vi "Gymkhana.vi"() -> ()   [LabVIEW 2020]
uses:
  Control/GymkhanaBestRecordIndicator.ctl
  Control/GymkhanaCurrentRecordIndicator.ctl
  Control/GymkhanaSubLoopState.ctl
  Control/GymkhanaFlag.ctl
  CommonControl/Flag.ctl
  Control/GymkhanaMainLoopState.ctl
  <vilib>/DAQmx/write.llb/DAQmx Write (Analog 1D DBL NChan 1Samp).vi
  <vilib>/DAQmx/read.llb/DAQmx Read (Analog 1D DBL NChan 1Samp).vi
  <vilib>/DAQmx/write.llb/DAQmx Write (Digital 1D Bool NChan 1Samp 1Line).vi
  <vilib>/DAQmx/create/channels.llb/DAQmx Create Channel (AO-Voltage-Basic).vi
  <vilib>/DAQmx/create/channels.llb/DAQmx Create Channel (AI-Voltage-Basic).vi
  <vilib>/DAQmx/create/channels.llb/DAQmx Create Channel (DO-Digital Output).vi
  <vilib>/DAQmx/miscellaneous.llb/DAQmx Fill In Error Info.vi
  <vilib>/Utility/file.llb/Write Delimited Spreadsheet (string).vi
panel:
  in  "GreenFlag":bool
  in  "RedFlag":bool
  in  "SignSignalDAQResources":tag
  out "GymkhanaFlag":T1
  out "Entry-B-InternalData":T3
  out "Entry-A-InternalData":T4
  in  "Entry-A-DNF":bool
  in  "Entry-B-DNF":bool
  out "CurrentRecordIndicator":T5
  out "BestRecordIndicator":T6
  in  "SensorDAQResources":tag
  in  "NextEntry":bool
  in  "Stop":bool
  # "2020 KSAE Formula Gymkhana Event"
  # "Time :"
  # "Time :"
  # "Entry :"
  # "Entry :"
  # "Univ. :"
  # "Univ. :"
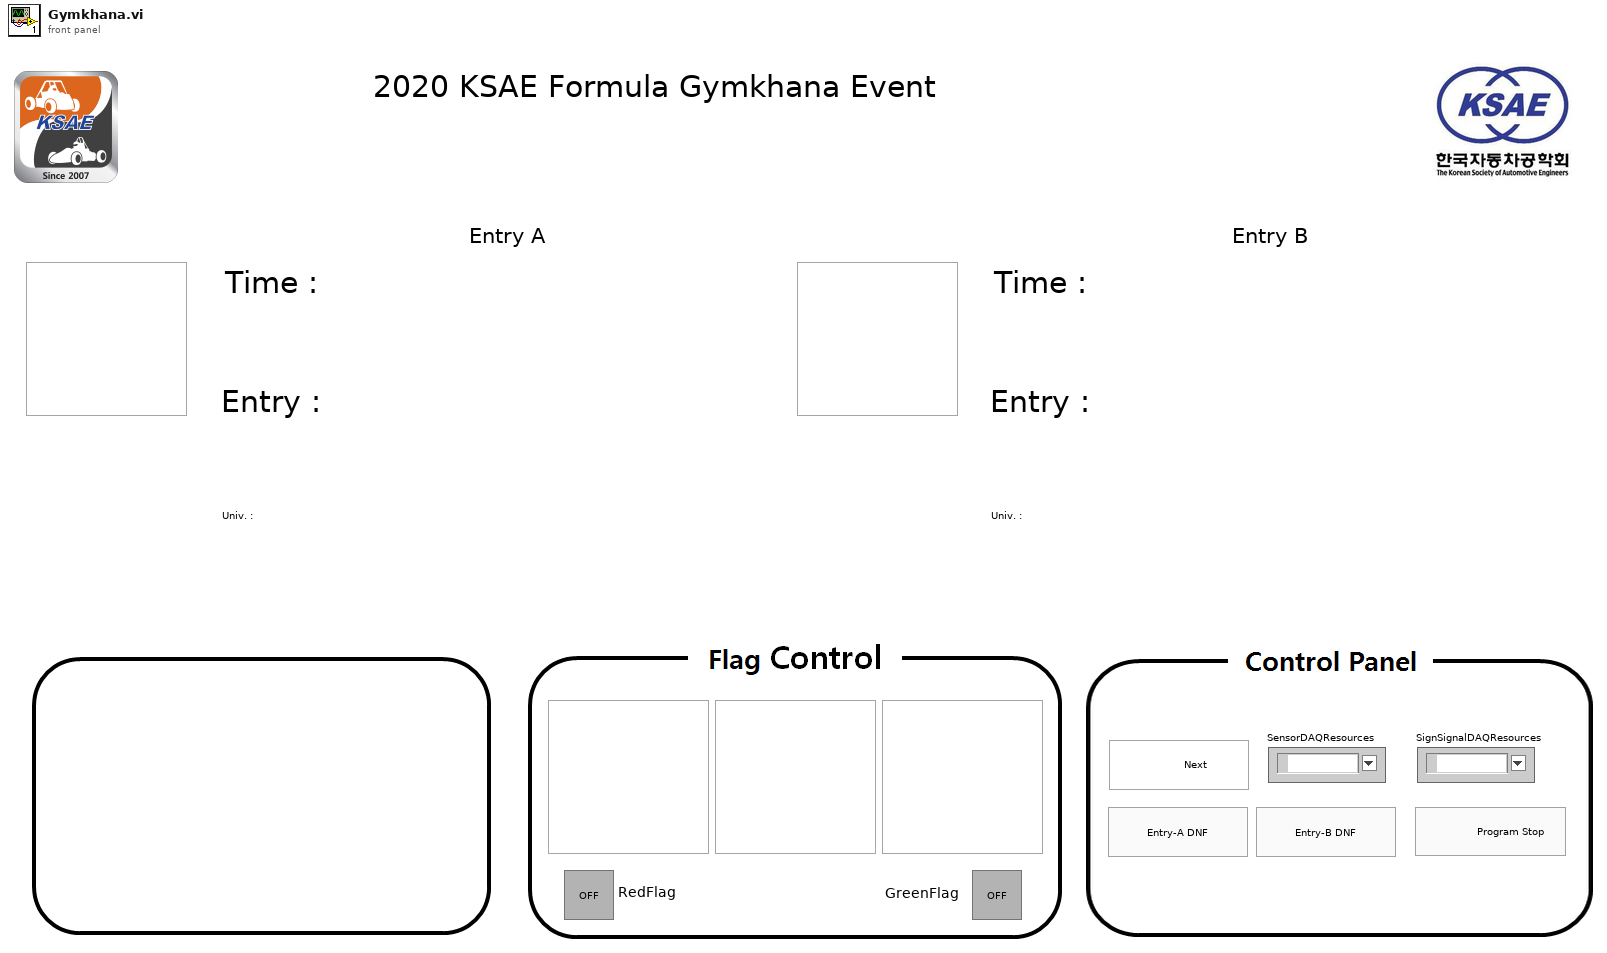
[diagram p1: front panel]
types:
  T1 = typedef "GymkhanaFlag.ctl" = cluster{"Red":picture, "Blank":picture, "Green":picture}
  T2 = typedef "GymkhanaSubLoopState.ctl" = enum16{"Initial", "Ready", "Running", "FinishRunning", "DNF"}
  T3 = cluster{"GymkhanaSubLooptate":T2, "Entry-B-RefTime(ms)":i64, "Entry-B-LabTime(ms)":i64}
  T4 = cluster{"GymkhanaSubloopState":T2, "Entry-ARefTime(ms)":i64, "Entry-ALabTime(ms)":i64}
  T5 = typedef "GymkhanaCurrentRecordIndicator.ctl" = cluster{"CurrentTime-A":string, "CurrentEntry-A":string, "CurrentUniversity-A":string, "Flag-A":picture, "CurrentMessage-A":string, "CurrentTime-B":string, "CurrentEntry-B":string, "CurrentUniversity-B":string, "Flag-B":picture, "CurrentMessage-B":string}
  T6 = typedef "GymkhanaBestRecordIndicator.ctl" = cluster{"BestTime":string, "BestEntry":string, "BestUniv":string}
  T7 = cluster{"StartEntry-B":bool, "PassLineEntry-B":bool, "NextEntry-B":bool, "DNFEntry-B":bool, "RetryEntry-B":bool}
  T8 = cluster{"GymkhanaSubloopState":T2, "Entry-A-RefTime(ms)":i64, "Entry-A-LabTime(ms)":i64}
  T9 = cluster{"StartEntry-A":bool, "PassLineEntry-A":bool, "NextEntry-A":bool, "DNFEntry-A":bool, "RetryEntry-A":bool}
  T10 = enum16{"open", "replace", "create", "open or create", "replace or create", "replace or create with confirmation"}
  T11 = typedef "Flag.ctl" = cluster{"GreenFlag":picture, "BlueFlag":picture, "RedFlag":picture, "CheckFlag":picture}
  T12 = typedef "GymkhanaMainLoopState.ctl" = enum16{"Initial", "InputInfomation", "Running", "RecordLog", "WaittingforNext", "ProgramStop"}
  T13 = cluster{"CurrentRecordIndicator":T5, "BestRecordIndicator":T6, "FlageData":T11, "LapTime-A(ms)":i64, "LapTime-B(ms)":i64, "StateValue":T12, "SignRedFlag":bool, "SignGreenFlag":bool, "Ready":bool, "NextEntry":bool, "DNFEntry-A":bool, "DNFEntry-B":bool, "RetryEntry-A":bool, "RetryEntry-B":bool, "Stop":bool}
  T14 = cluster{"CurrentEntry":string, "CurrentUniv":string, "CurrentTeam":string, "DNF":bool}[]
  T15 = cluster{"CurrentEntry":string, "CurrentUniv":string, "CurrentTeam":string, "DNF":bool}
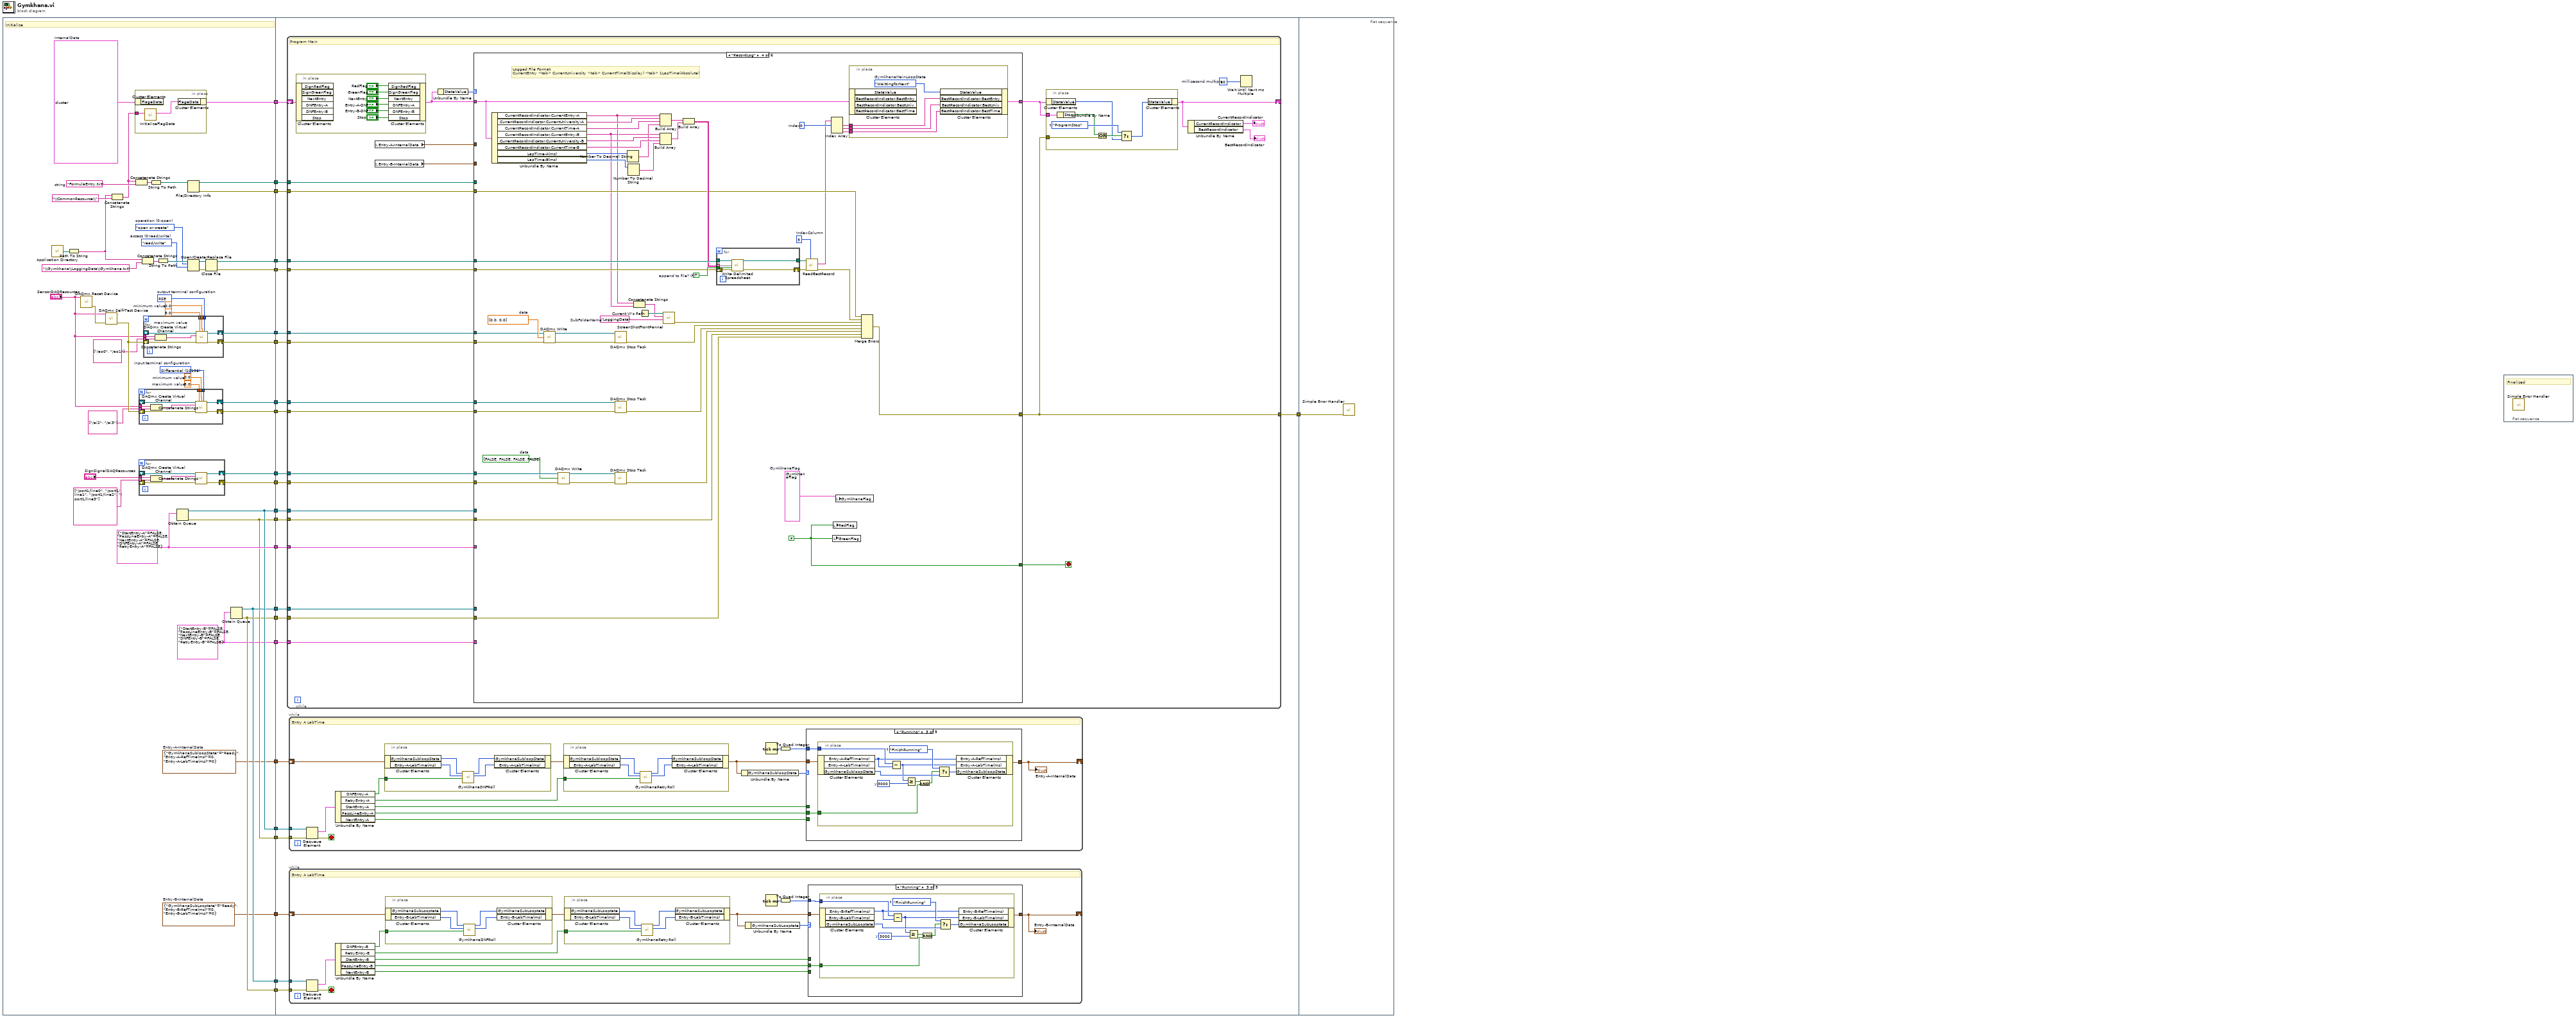
[diagram p0: block diagram]
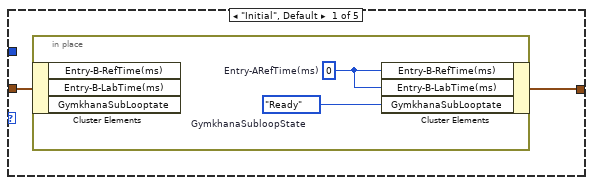
[diagram p2: hidden frame]
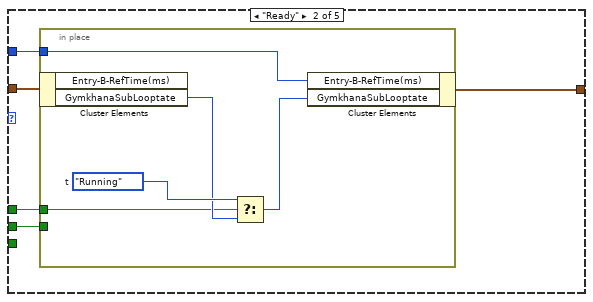
[diagram p3: hidden frame]
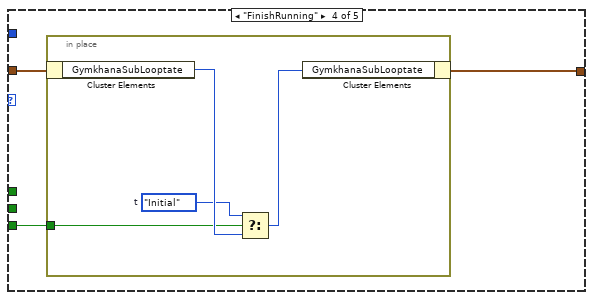
[diagram p4: hidden frame]
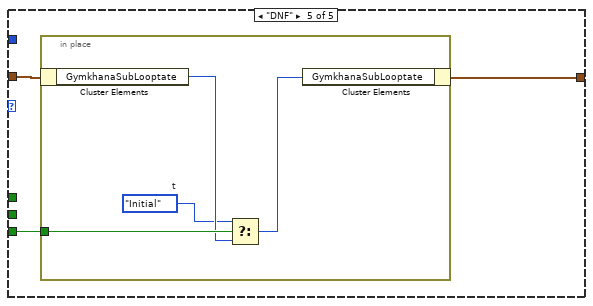
[diagram p5: hidden frame]
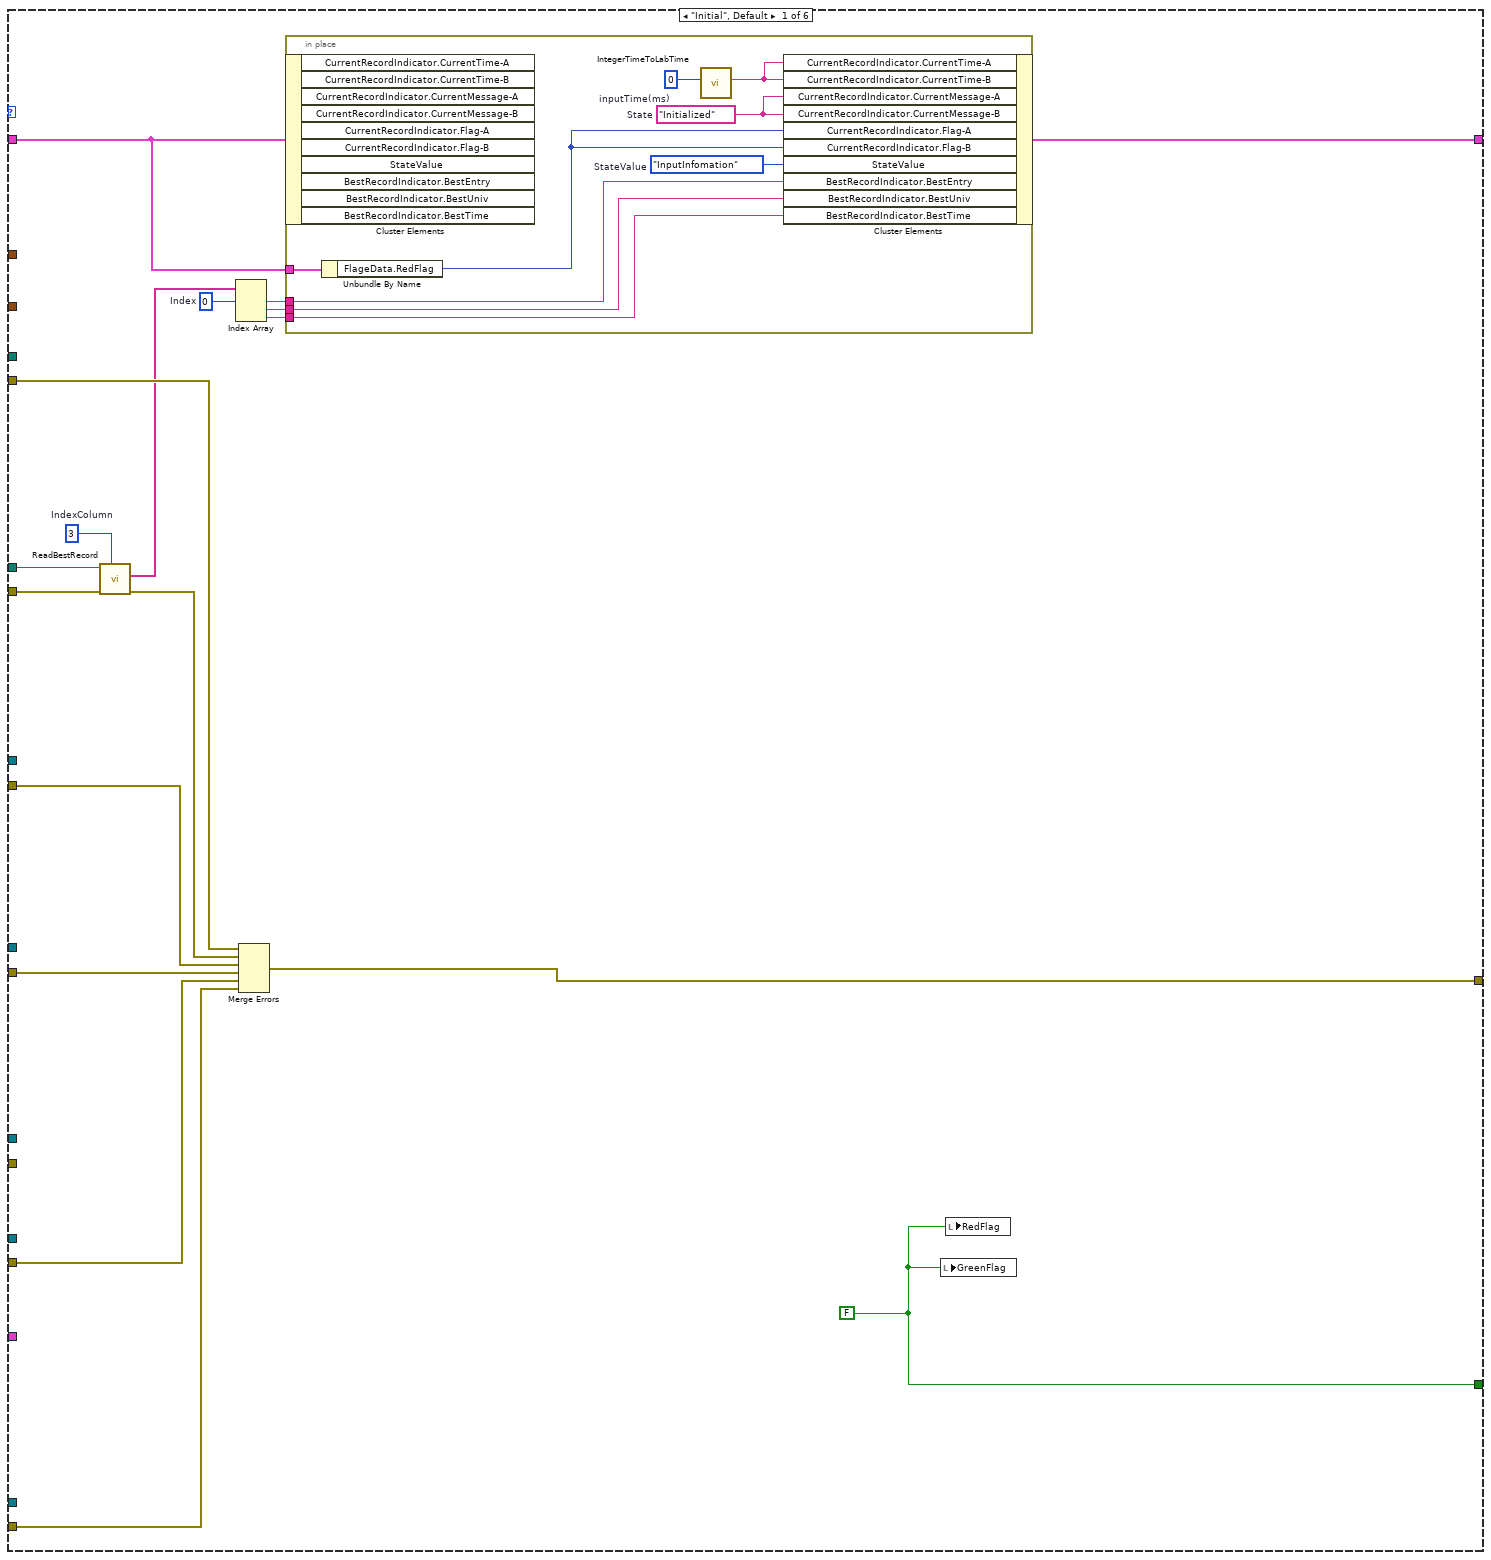
[diagram p6: hidden frame]
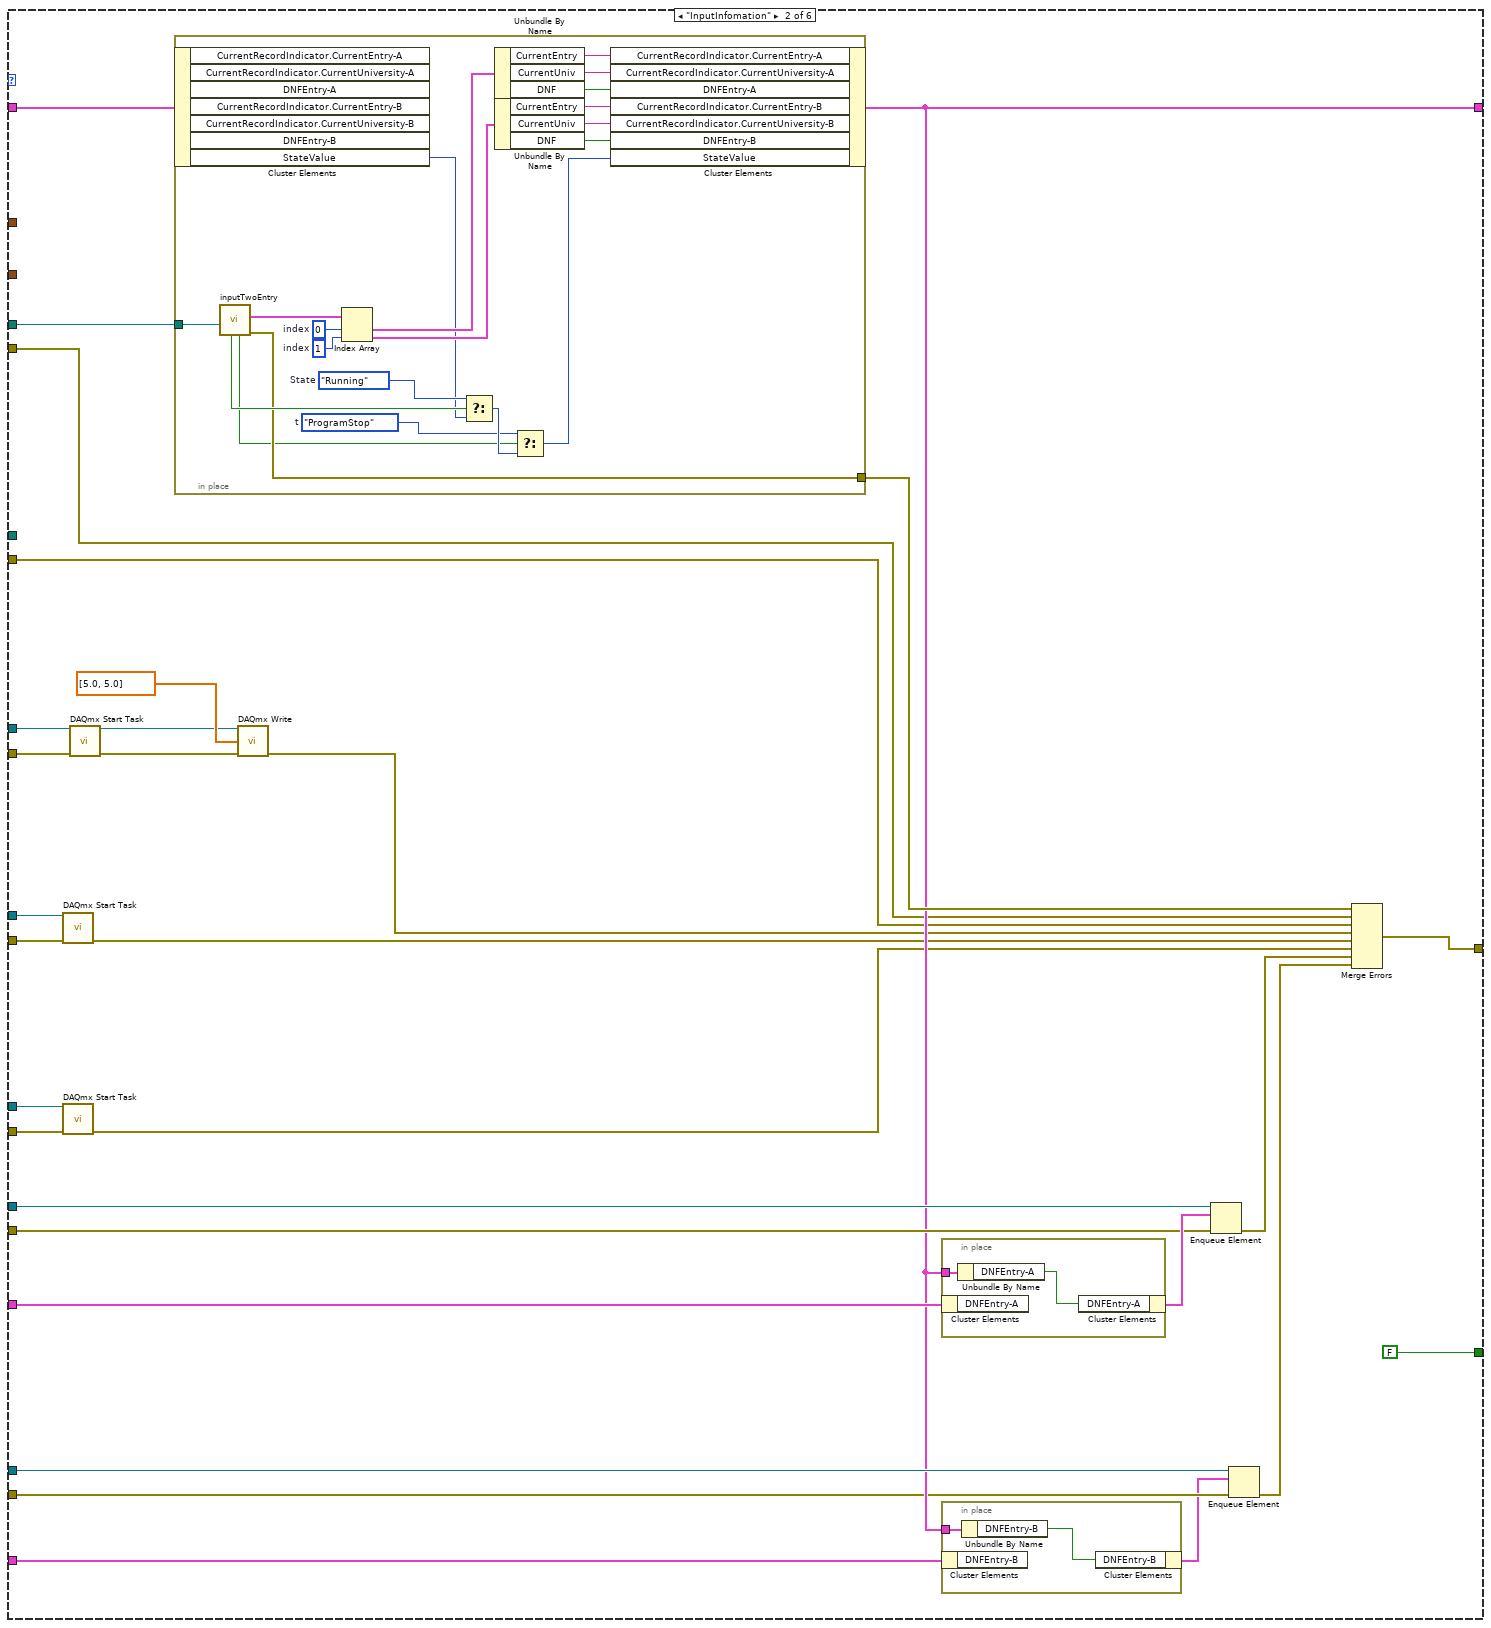
[diagram p7: hidden frame]
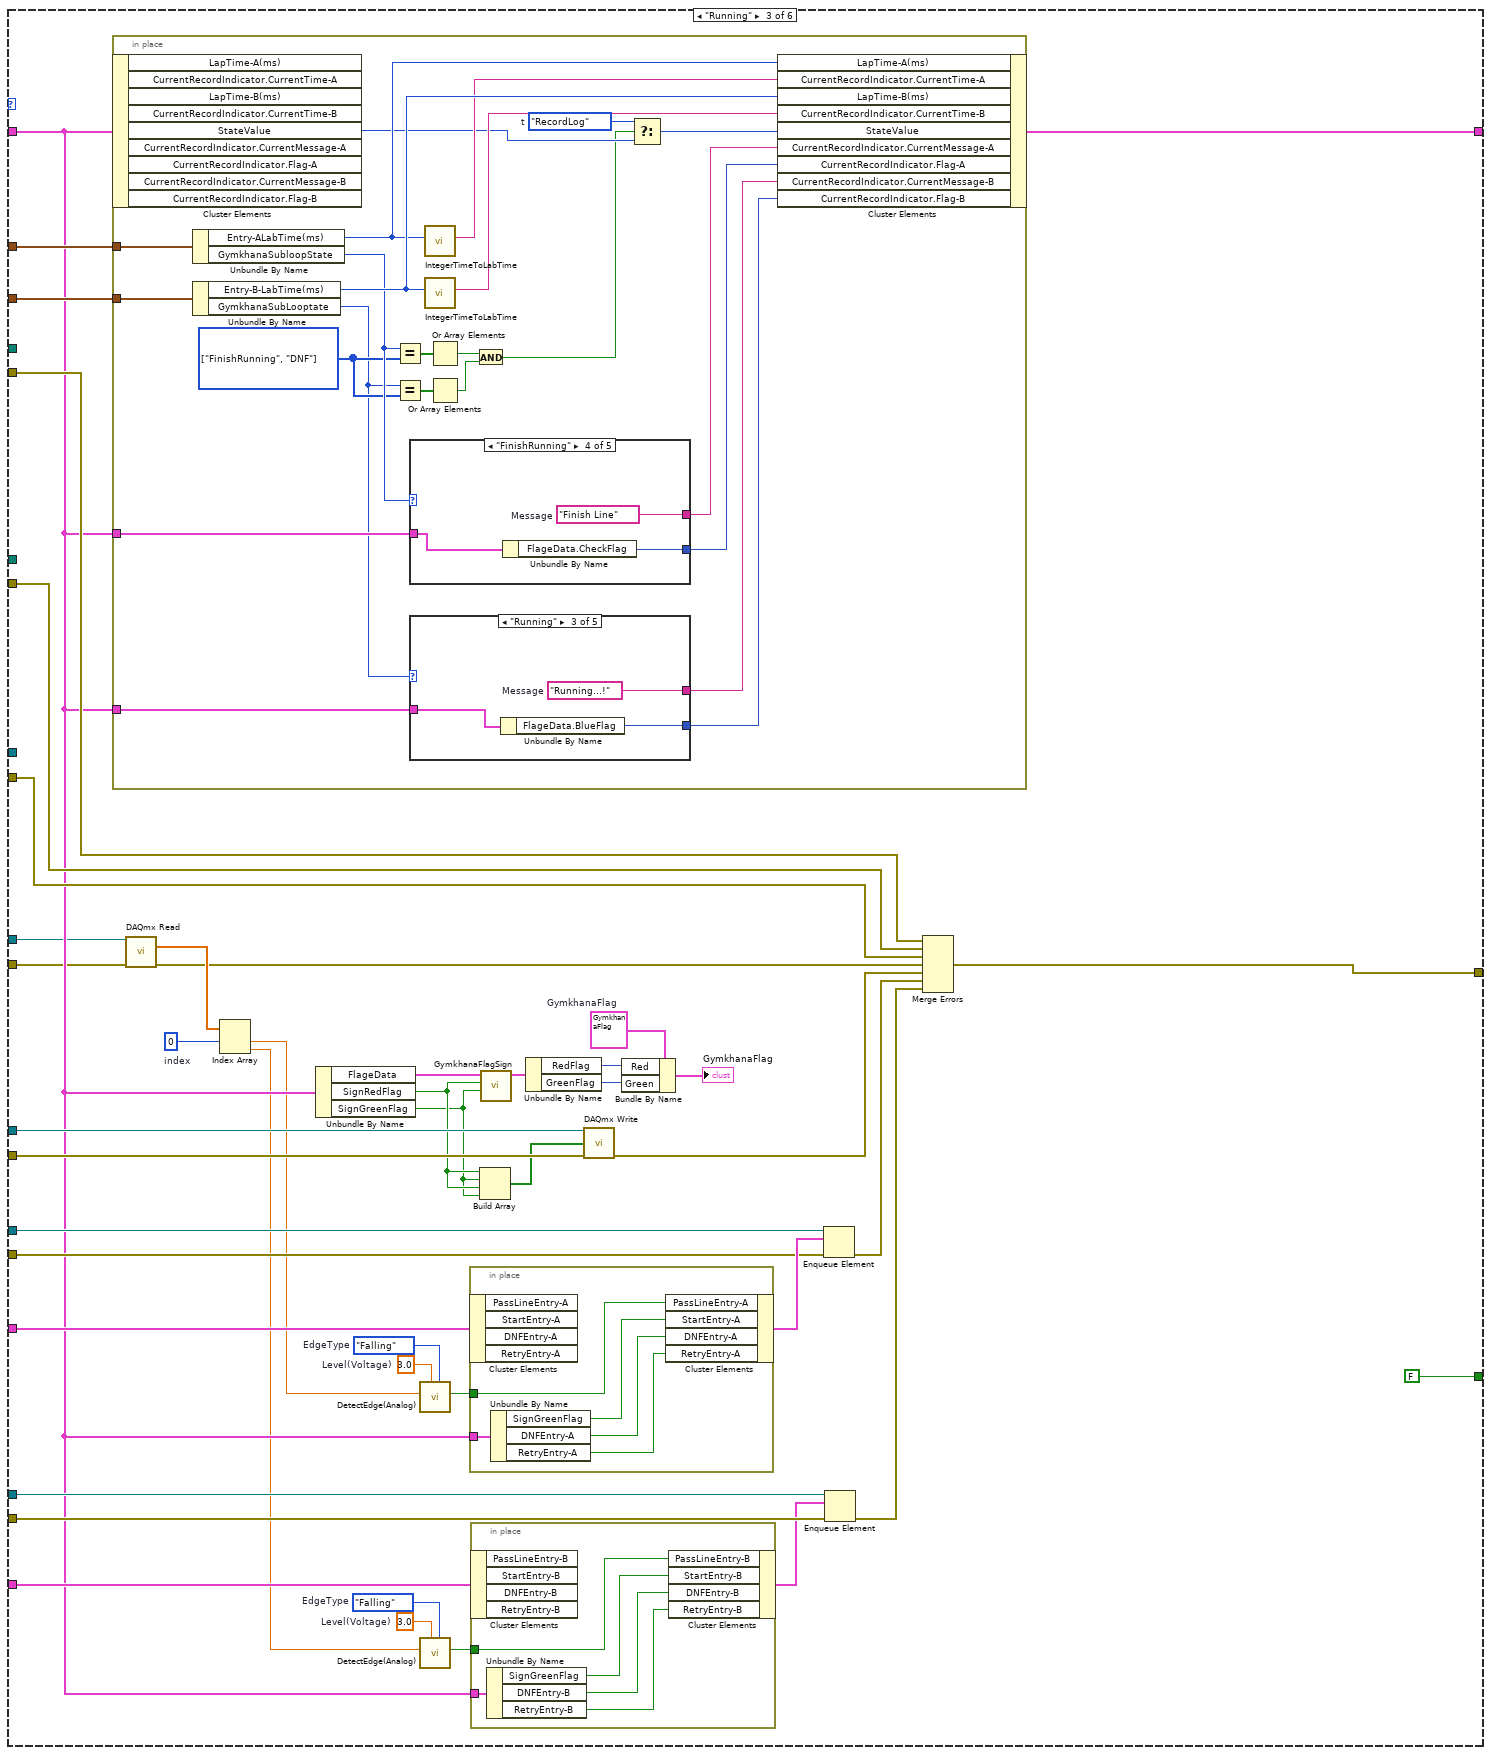
[diagram p8: hidden frame]
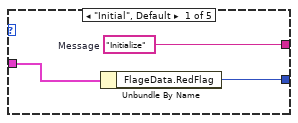
[diagram p9: hidden frame]
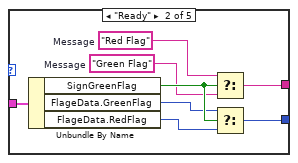
[diagram p10: hidden frame]
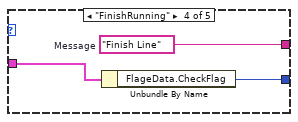
[diagram p11: hidden frame]
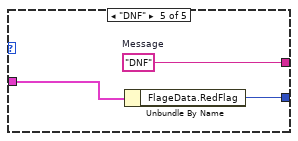
[diagram p12: hidden frame]
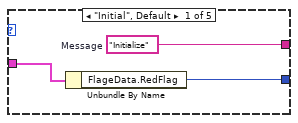
[diagram p13: hidden frame]
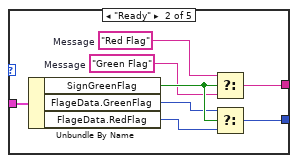
[diagram p14: hidden frame]
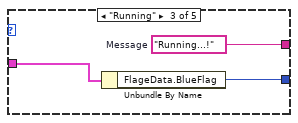
[diagram p15: hidden frame]
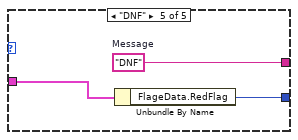
[diagram p16: hidden frame]
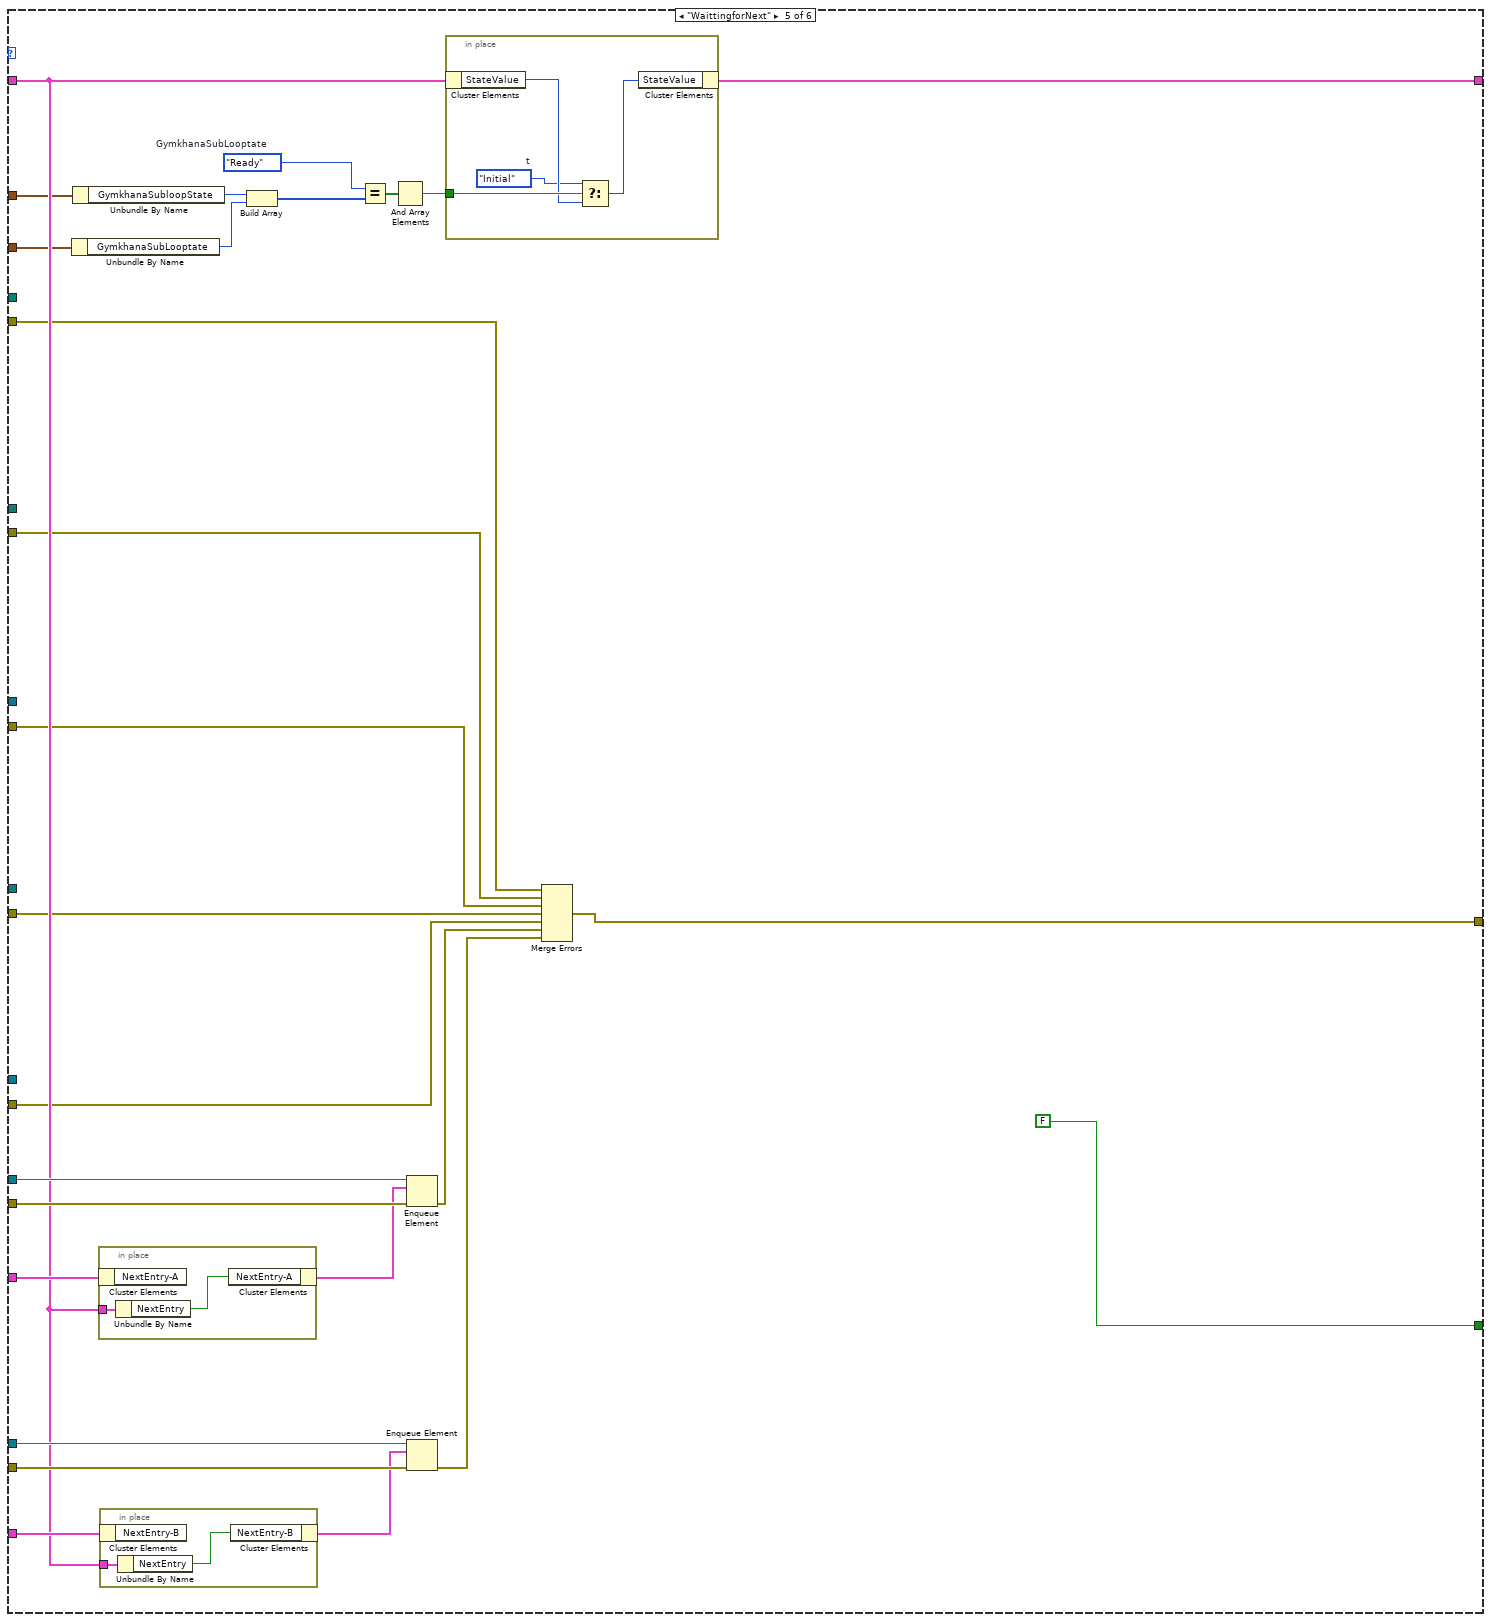
[diagram p17: hidden frame]
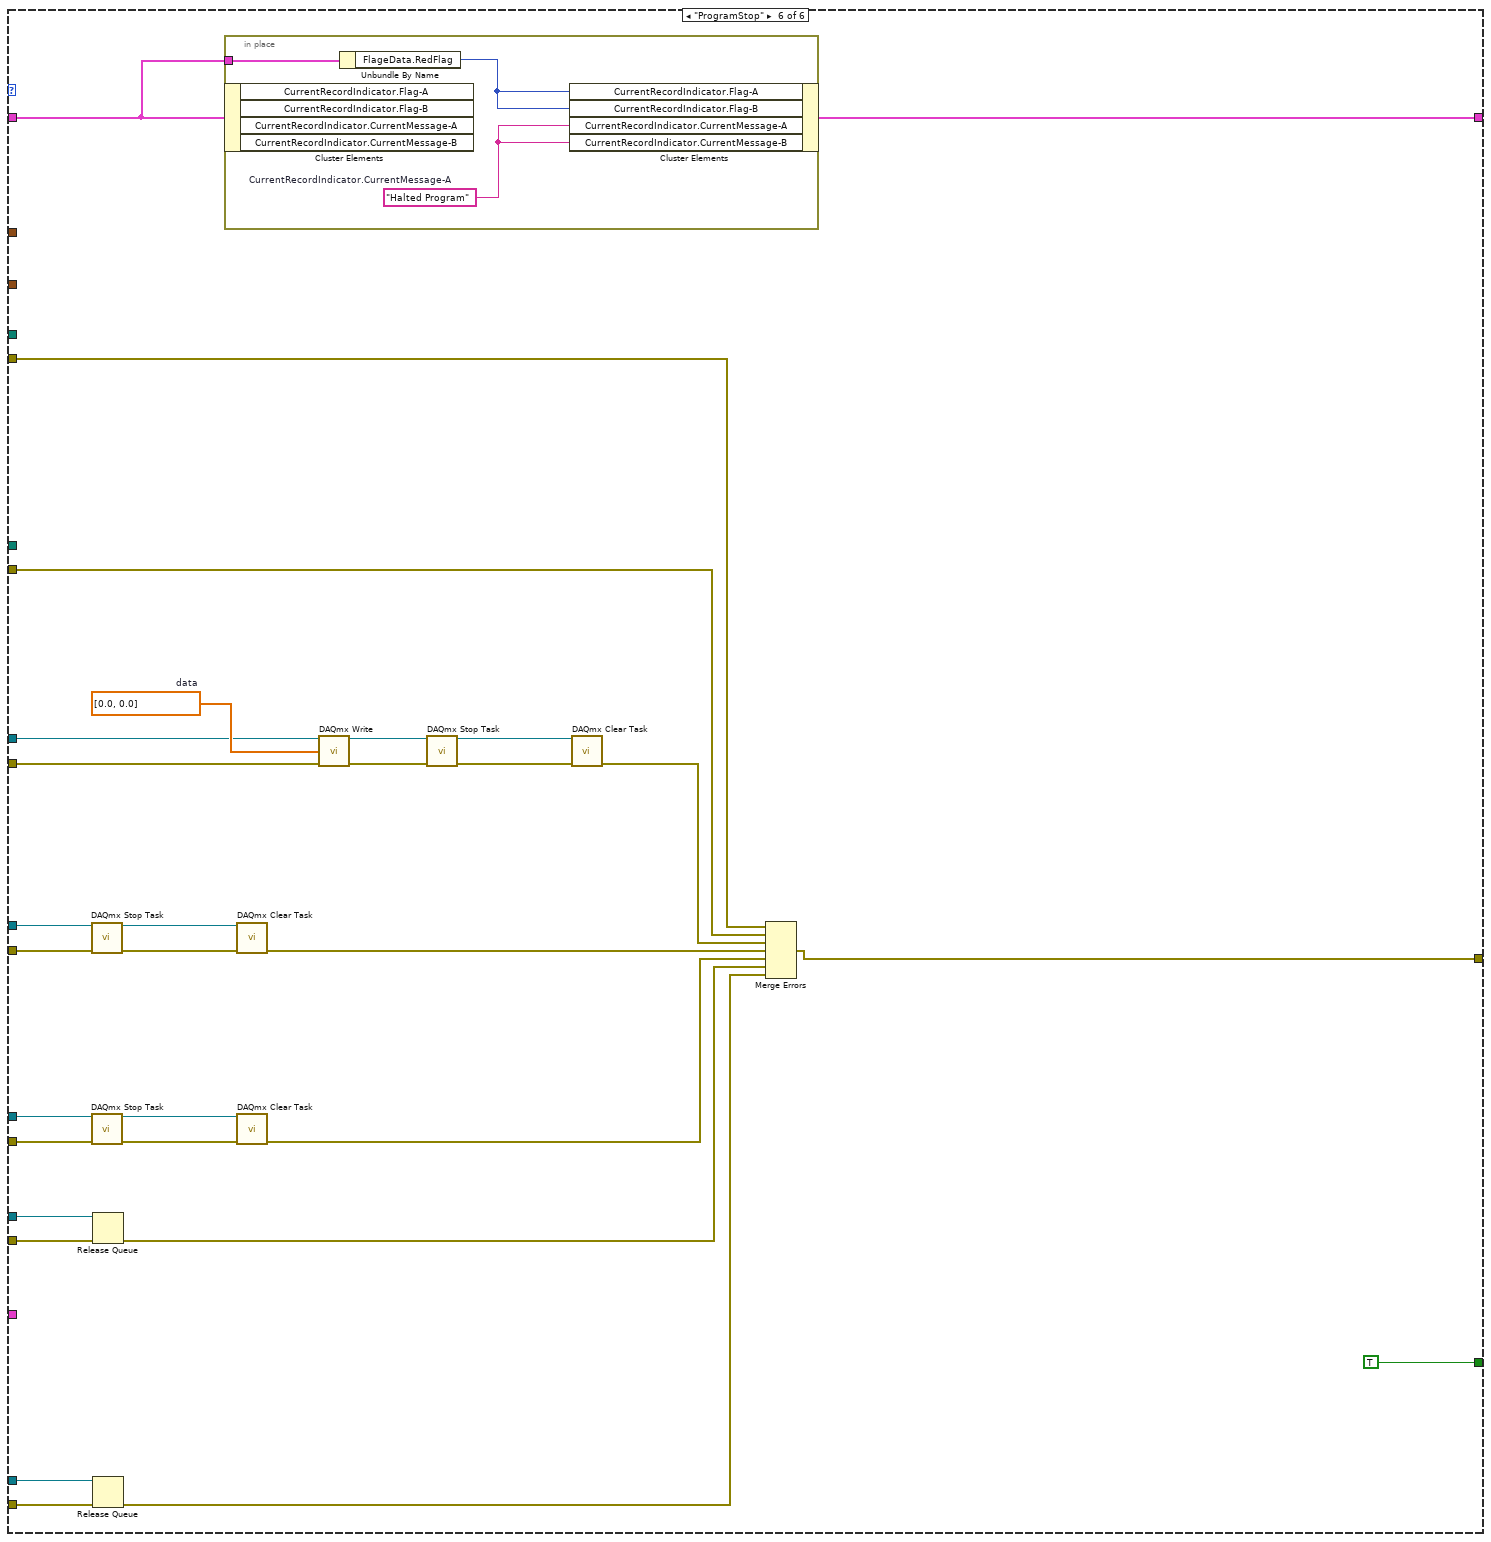
[diagram p18: hidden frame]
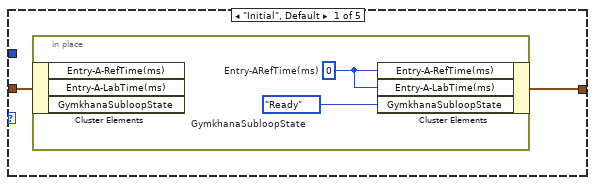
[diagram p19: hidden frame]
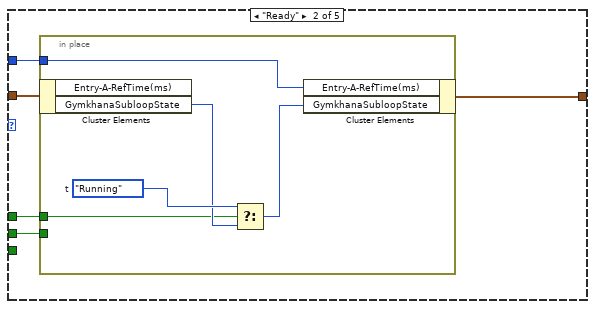
[diagram p20: hidden frame]
diagram:
  n1 = flat-sequence {
    tunnel: [w56] -> w24
    tunnel: [w47] -> w23
    tunnel: [w39] -> w22
    tunnel: [w52] -> w21
    tunnel: [w49] -> w20
    tunnel: [w43] -> w19
    tunnel: [w42] -> w18
    tunnel: [w44] -> w17
    tunnel: [w34] -> w16
    tunnel: [w43] -> w15
    tunnel: [w42] -> w14
    tunnel: [w41] -> w13
    tunnel: [w40] -> w12
    tunnel: [w41] -> w11
    tunnel: [w40] -> w10
    tunnel: [w33] -> w8
    tunnel: [w32] -> w7
    tunnel: [w31] -> w6
    tunnel: [w30] -> w5
    tunnel: [w36] -> w4
    tunnel: [w35] -> w3
    tunnel: [w27] -> w2
    tunnel: [w26] -> w1
    tunnel: w24 -> [w124]
    tunnel: w23 -> [w123]
    tunnel: w22 -> [w122]
    tunnel: w21 -> [w119]
    tunnel: w20 -> [w121]
    tunnel: w19 -> [w120]
    tunnel: w18 -> [w118]
    tunnel: w17 -> [w117]
    tunnel: w16 -> [w116]
    tunnel: w15 -> [w115]
    tunnel: w14 -> [w103]
    tunnel: w13 -> [w114]
    tunnel: w12 -> [w113]
    tunnel: w11 -> [w112]
    tunnel: w10 -> [w104]
    tunnel: [w111] -> w9
    tunnel: w8 -> [w110]
    tunnel: w7 -> [w109]
    tunnel: w6 -> [w108]
    tunnel: w5 -> [w107]
    tunnel: w4 -> [w106]
    tunnel: w3 -> [w105]
    tunnel: w2 -> [w102]
    tunnel: w1 -> [w101]
    tunnel: w9 -> [w630]
    frame #0 {
      w34 = T7 {"StartEntry-B"=FALSE, "PassLineEntry-B"=FALSE, "NextEntry-B"=FALSE, "DNFEntry-B"=FALSE, "RetryEntry-B"=FALSE}
      w35 = T3 {"GymkhanaSubLooptate"=enum."Ready", "Entry-B-RefTime(ms)"=0, "Entry-B-LabTime(ms)"=0}  # Entry-B-InternalData
      w36 = T8 {"GymkhanaSubloopState"=enum."Ready", "Entry-A-RefTime(ms)"=0, "Entry-A-LabTime(ms)"=0}  # Entry-A-InternalData
      w44 = T9 {"StartEntry-A"=FALSE, "PassLineEntry-A"=FALSE, "NextEntry-A"=FALSE, "DNFEntry-A"=FALSE, "RetryEntry-A"=FALSE}
      w45 = enum16{"read/write", "read-only", "write-only"}."read/write"  # access (0:read/write)
      w46 = T10."open or create"  # operation (0:open)
      w55 = 5.0  # maximum value
      w54 = 0.0  # minimum value
      w53 = 10106 items=["default"=-1, "RSE"=10083, "NRSE"=10078, "Differential"=10106, "Pseudodifferential"=12529]  # input terminal configuration
      w38 = T13 {"CurrentRecordIndicator"={"CurrentTime-A"="", "CurrentEntry-A"="", "CurrentUniversity-A"="", "Flag-A"=bytes[0], "CurrentMessage-A"="", "CurrentTime-B"="", "CurrentEntry-B"="", "CurrentUniversity-B"="", "Flag-B"=bytes[0], "CurrentMessage-B"=""}, "BestRecordIndicator"={"BestTime"="", "BestEntry"="", "BestUniv"=""}, "FlageData"={"GreenFlag"=bytes[0], "BlueFlag"=bytes[0], "RedFlag"=bytes[0], "CheckFlag"=bytes[0]}, "LapTime-A(ms)"=0, "LapTime-B(ms)"=0, "StateValue"=enum."Initial", "SignRedFlag"=FALSE, "SignGreenFlag"=FALSE, "Ready"=FALSE, "NextEntry"=FALSE, "DNFEntry-A"=FALSE, "DNFEntry-B"=FALSE, "RetryEntry-A"=FALSE, "RetryEntry-B"=FALSE, "Stop"=FALSE}  # InternalData
      w62 = "FormulaEntry.txt"  # string
      w69 = 10083 items=["Default"=-1, "RSE"=10083, "Differential"=10106, "Pseudodifferential"=12529]  # output terminal configuration
      w70 = 0.0  # minimum value
      w71 = 5.0  # maximum value
      # "Initialize"
      n2 = call <vilib>:"Application Directory.vi"() -> ("Application Directory"=w68:path)
      n3 = Path To String(path=w68) -> (string=w64:string)
      n4 = call <vilib>:"DAQmx Reset Device.vi"("device in"="SensorDAQResources") -> ("error out"=w60:errorcluster)  [unwired: 14 in]
      n5 = call <vilib>:"DAQmx Self-Test Device.vi"("device in"="SensorDAQResources", "error in"=w60) -> ("error out"=w59:errorcluster)  [unwired: 13 in]
      n6 = Concatenate Strings "Concatenate Strings"(w64, "\\CommonResource\\") -> (w37:string)
      n7 = in-place {
        in-place-border: w37 -> [w80]
        n8 = in-place-cluster #1(w38) -> ()  [unwired: 1 out]
        n9 = call "InitializeFlagData.vi"("inputPath"=w80) -> ("outputFlagData"=w79:T11)  [unwired: 9 in, 1 out]
        n10 = in-place-cluster #1("FlageData"=w79) -> (w39:T13)
      }
      n11 = Concatenate Strings "Concatenate Strings"(w37, w62) -> (w63:string)
      n12 = for {
        shift-right: [w89] -> w30
        shift-left: w59 -> [w88]
        tunnel: string[] ["/ai2", "/ai3"] -> [w87] mode=indexing
        shift-right: [w90] -> w31
        shift-left: _ -> [w86]
        tunnel: "SensorDAQResources" -> [w85]
        tunnel: w55 -> [w84]
        tunnel: w54 -> [w83]
        tunnel: w53 -> [w82]
        n13 = Concatenate Strings(w85, w87) -> (w81:string)
        n14 = call-poly <vilib>:"DAQmx Create Virtual Channel.vi"("task in"=w86, "maximum value"=w84, "minimum value"=w83, "input terminal configuration"=w82, "physical channels"=w81, "error in"=w88) -> ("task out"=w90:refnum<k21>, "error out"=w89:errorcluster)  [unwired: 8 in]
      }
      n15 = for {
        shift-right: [w77] -> w26
        shift-left: _ -> [w76]
        tunnel: string[] ["/port1/line0", "/port1/line1", "/port1/line2", "/port1/line3"] -> [w75] mode=indexing
        shift-right: [w78] -> w27
        shift-left: _ -> [w74]
        tunnel: "SignSignalDAQResources" -> [w73]
        n16 = Concatenate Strings(w73, w75) -> (w72:string)
        n17 = call-poly <vilib>:"DAQmx Create Virtual Channel.vi"("task in"=w74, "lines"=w72, "error in"=w76) -> ("task out"=w78:refnum<k21>, "error out"=w77:errorcluster)  [unwired: 11 in]
      }
      n18 = Concatenate Strings "Concatenate Strings"(w64, "\\Gymkhana\\LoggingData\\Gymkhana.txt") -> (w66:string)
      n19 = for {
        tunnel: w71 -> [w99]
        tunnel: w70 -> [w98]
        tunnel: w69 -> [w97]
        tunnel: "SensorDAQResources" -> [w93]
        shift-right: [w95] -> w32
        shift-left: w59 -> [w94]
        tunnel: string[] ["/ao0", "/ao1"] -> [w92] mode=indexing
        shift-right: [w100] -> w33
        shift-left: _ -> [w91]
        n20 = Concatenate Strings(w93, w92) -> (w96:string)
        n21 = call-poly <vilib>:"DAQmx Create Virtual Channel.vi"("task in"=w91, "maximum value"=w99, "minimum value"=w98, "output terminal configuration"=w97, "physical channels"=w96, "error in"=w94) -> ("task out"=w100:refnum<k21>, "error out"=w95:errorcluster)  [unwired: 8 in]
      }
      n22 = String To Path(string=w63) -> (path=w61:path)
      n23 = String To Path(string=w66) -> (path=w51:path)
      n24 = Obtain Queue(element data type=w44) -> (queue out=w43:refnum<queue>, error out=w41:errorcluster)  [unwired: 4 in, 1 out]
      n25 = Open/Create/Replace File(file path (use dialog)=w51, operation (0:open)=w46, access (0:read/write)=w45) -> (refnum out=w50:refnum<file>, error out=w48:errorcluster)  [unwired: 3 in, 1 out]
      n26 = File/Directory Info(path=w61) -> (path out=w56:path, error out=w52:errorcluster)  [unwired: 1 in, 5 out]
      n27 = Close File(refnum=w50, error in=w48) -> (path=w49:path, error out=w47:errorcluster)
      n28 = Obtain Queue(element data type=w34) -> (queue out=w42:refnum<queue>, error out=w40:errorcluster)  [unwired: 4 in, 1 out]
    }
    frame #1 {
      n29 = while {
        shift-right: [w202] -> _
        shift-left: w122 -> [w198]
        tunnel: w124 -> [w204]
        tunnel: w123 -> [w211]
        tunnel: w121 -> [w218]
        tunnel: w120 -> [w217]
        tunnel: w119 -> [w203]
        tunnel: w118 -> [w216]
        tunnel: w117 -> [w215]
        tunnel: w116 -> [w214]
        tunnel: w114 -> [w213]
        tunnel: w113 -> [w212]
        tunnel: [w199] -> w111
        tunnel: w110 -> [w209]
        tunnel: w109 -> [w208]
        tunnel: w108 -> [w207]
        tunnel: w107 -> [w206]
        tunnel: w102 -> [w194]
        tunnel: w101 -> [w193]
        stop <- w205 stop-if-true
        w220 = u32 10  # millisecond multiple
        # "Program Main"
        n30 = in-place {
          n31 = in-place-cluster #2(w198) -> ()  [unwired: 6 out]
          n32 = in-place-cluster #2("SignRedFlag"="RedFlag", "SignGreenFlag"="GreenFlag", "NextEntry"="NextEntry", "DNFEntry-A"="Entry-A-DNF", "DNFEntry-B"="Entry-B-DNF", "Stop"="Stop") -> (w195:T13)
        }
        n33 = local read "Entry-A-InternalData"() -> (w201:T4)
        n34 = local read "Entry-B-InternalData"() -> (w200:T3)
        n35 = Unbundle By Name(w195) -> ("StateValue"=w197:T12)
        n36 = case shown="\"RecordLog\"" w197 {
          tunnel: w195 -> [w243 w283 w323 w442 w500 w545]
          tunnel: [w244 w268 w349 w443 w506 w546] -> w196
          tunnel: w218 -> [w234 _ _ w472 _ _]
          tunnel: w217 -> [_ w276 w351 _ w513 w551]
          tunnel: w216 -> [_ w275 w350 _ w511 w549]
          tunnel: w215 -> [_ w274 w348 _ w505 _]
          tunnel: w214 -> [_ w271 w331 _ w504 _]
          tunnel: w213 -> [w242 w270 w346 w466 w512 w550]
          tunnel: w212 -> [w241 w267 w345 w465 w510 w548]
          tunnel: w211 -> [w235 w254 w333 w473 w488 w528]
          tunnel: [w240 w281 w342 w464 w507 w531] -> w199
          tunnel: w209 -> [_ w277 _ w450 _ w530]
          tunnel: w208 -> [w228 w264 w328 w451 w495 w529]
          tunnel: w207 -> [_ w258 w316 w446 _ w534]
          tunnel: w206 -> [w229 w259 w315 w445 w494 w535]
          tunnel: [w227 FALSE FALSE w425 FALSE TRUE] -> w205
          tunnel: w204 -> [_ w279 _ _ _ _]
          tunnel: w203 -> [w239 w255 w332 w456 w493 w527]
          tunnel: w201 -> [_ _ w340 _ w499 _]
          tunnel: w200 -> [_ _ w339 _ w498 _]
          tunnel: w194 -> [_ w262 w327 w430 _ w524]
          tunnel: w193 -> [_ w261 w326 w429 w487 w523]
          frame "Initial", Default {
            w238 = 3  # IndexColumn
            w237 = 0  # Index
            w227 = FALSE
            n37 = call "ReadBestRecord.vi"("IndexColumn"=w238, "ErrorInput"=w235, "FilepathInput"=w234) -> ("ErrorOutput"=w233:errorcluster, "Data"=w236:string[])  [unwired: 6 in, 1 out]
            n38 = Index Array "Index Array"(array=w236, index #1=w237) -> (element #1=w232:string, element #2=w231:string, element #3=w230:string)  [unwired: 2 in]
            n39 = Merge Errors "Merge Errors"(w239, w233, w228, w229, w242, w241) -> (w240:errorcluster)
            n40 = in-place {
              in-place-border: w243 -> [w253]
              in-place-border: w232 -> [w247]
              in-place-border: w231 -> [w246]
              in-place-border: w230 -> [w245]
              w248 = GymkhanaMainLoopState."InputInfomation"  # StateValue
              w251 = i64 0  # inputTime(ms)
              w249 = "Initialized"  # State
              n41 = in-place-cluster #3(w243) -> ()  [unwired: 10 out]
              n42 = Unbundle By Name(w253) -> ("FlageData.RedFlag"=w252:picture)
              n43 = call "IntegerTimeToLabTime.vi"("inputTime(msec)"=w251) -> ("outputTime(mm-ss-sss)"=w250:string)  [unwired: 10 in]
              n44 = in-place-cluster #3("CurrentRecordIndicator.CurrentTime-A"=w250, "CurrentRecordIndicator.CurrentTime-B"=w250, "CurrentRecordIndicator.CurrentMessage-A"=w249, "CurrentRecordIndicator.CurrentMessage-B"=w249, "CurrentRecordIndicator.Flag-A"=w252, "CurrentRecordIndicator.Flag-B"=w252, "StateValue"=w248, "BestRecordIndicator.BestEntry"=w247, "BestRecordIndicator.BestUniv"=w246, "BestRecordIndicator.BestTime"=w245) -> (w244:T13)
            }
            n45 = local write "GreenFlag"(w227) -> ()
            n46 = local write "RedFlag"(w227) -> ()
          }
          frame "InputInfomation" {
            n47 = call <vilib>:"DAQmx Start Task.vi"("task/channels in"=w258, "error in"=w259) -> ("error out"=w257:errorcluster)  [unwired: 12 in, 1 out]
            n48 = call <vilib>:"DAQmx Start Task.vi"("task/channels in"=w262, "error in"=w261) -> ("error out"=w260:errorcluster)  [unwired: 12 in, 1 out]
            n49 = call <vilib>:"DAQmx Start Task.vi"("task/channels in"=w277, "error in"=w264) -> ("task out"=w265:refnum<k21>, "error out"=w263:errorcluster)  [unwired: 12 in]
            n50 = in-place {
              in-place-border: w279 -> [w300]
              in-place-border: [w293] -> w282
              w295 = GymkhanaMainLoopState."ProgramStop"  # t
              w298 = GymkhanaMainLoopState."Running"  # State
              w305 = 1  # index
              w306 = 0  # index
              n51 = in-place-cluster #4(w283) -> ("StateValue"=w297:T12)  [unwired: 6 out]
              n52 = call "inputTwoEntry.vi"("inputFilePath"=w300) -> ("ErrorOutput"=w293:errorcluster, "OutputData"=w307:T14, "StopButtonOutput"=w292:bool, "OKButtonOutput"=w299:bool)  [unwired: 7 in]
              n53 = Index Array(array=w307, index #1=w306, index #2=w305) -> (element #1=w304:T15, element #2=w302:T15)
              n54 = Select(t=w298, s=w299, f=w297) -> (s? t:f=w296:T12)
              n55 = Unbundle By Name(w304) -> ("CurrentEntry"=w291:string, "CurrentUniv"=w303:string, "DNF"=w289:bool)
              n56 = Unbundle By Name(w302) -> ("CurrentEntry"=w290:string, "CurrentUniv"=w301:string, "DNF"=w288:bool)
              n57 = Select(t=w295, s=w292, f=w296) -> (s? t:f=w294:T12)
              n58 = in-place-cluster #4("CurrentRecordIndicator.CurrentEntry-A"=w291, "CurrentRecordIndicator.CurrentUniversity-A"=w303, "DNFEntry-A"=w289, "CurrentRecordIndicator.CurrentEntry-B"=w290, "CurrentRecordIndicator.CurrentUniversity-B"=w301, "DNFEntry-B"=w288, "StateValue"=w294) -> (w268:T13)
            }
            n59 = call-poly <vilib>:"DAQmx Write.vi"("task/channels in"=w265, "data"=dbl[] [5.0, 5.0], "error in"=w263) -> ("error out"=w256:errorcluster)  [unwired: 10 in, 2 out]
            n60 = in-place {
              in-place-border: w268 -> [w287]
              n61 = in-place-cluster #5(w274) -> ()  [unwired: 1 out]
              n62 = Unbundle By Name(w287) -> ("DNFEntry-A"=w286:bool)
              n63 = in-place-cluster #5("DNFEntry-A"=w286) -> (w272:T9)
            }
            n64 = in-place {
              in-place-border: w268 -> [w285]
              n65 = in-place-cluster #6(w271) -> ()  [unwired: 1 out]
              n66 = Unbundle By Name(w285) -> ("DNFEntry-B"=w284:bool)
              n67 = in-place-cluster #6("DNFEntry-B"=w284) -> (w266:T7)
            }
            n68 = Enqueue Element(queue=w276, element=w272, error in (no error)=w270) -> (error out=w273:errorcluster)  [unwired: 1 in, 2 out]
            n69 = Enqueue Element(queue=w275, element=w266, error in (no error)=w267) -> (error out=w269:errorcluster)  [unwired: 1 in, 2 out]
            n70 = Merge Errors "Merge Errors"(w282, w255, w254, w256, w257, w260, w273, w269) -> (w281:errorcluster)
          }
          frame "Running" {
            w311 = 0  # index
            w320 = T1 {"Red"=bytes[0], "Blank"=bytes[0], "Green"=bytes[0]}  # GymkhanaFlag
            w334 = enum16{"Rising", "Falling"}."Falling"  # EdgeType
            w335 = enum16{"Rising", "Falling"}."Falling"  # EdgeType
            w337 = 3.0  # Level(Voltage)
            w338 = 3.0  # Level(Voltage)
            n71 = in-place {
              in-place-border: w340 -> [w384]
              in-place-border: w339 -> [w383]
              in-place-border: w323 -> [w372]
              in-place-border: w323 -> [w363]
              w368 = T2[] [enum."FinishRunning", enum."DNF"] items=["Initial", "Ready", "Running", "FinishRunning", "DNF"]
              w381 = GymkhanaMainLoopState."RecordLog"  # t
              n72 = in-place-cluster #7(w323) -> ("StateValue"=w376:T12)  [unwired: 8 out]
              n73 = Unbundle By Name(w384) -> ("Entry-ALabTime(ms)"=w378:i64, "GymkhanaSubloopState"=w371:T2)
              n74 = Unbundle By Name(w383) -> ("Entry-B-LabTime(ms)"=w380:i64, "GymkhanaSubLooptate"=w365:T2)
              n75 = Equal?(x=w371, y=w368) -> (x = y?=w369:bool[])
              n76 = Equal?(x=w365, y=w368) -> (x = y?=w367:bool[])
              n77 = case shown="\"FinishRunning\"" w371 {
                tunnel: [w407 w412 w418 w421 w424] -> w374
                tunnel: w372 -> [w406 w415 w417 w420 w423]
                tunnel: [w405 w409 w416 w419 w422] -> w373
                frame "Initial", Default {
                  w407 = "Initialize"  # Message
                  n78 = Unbundle By Name(w406) -> ("FlageData.RedFlag"=w405:picture)
                }
                frame "Ready" {
                  w408 = "Green Flag"  # Message
                  w414 = "Red Flag"  # Message
                  n79 = Unbundle By Name(w415) -> ("SignGreenFlag"=w413:bool, "FlageData.GreenFlag"=w411:picture, "FlageData.RedFlag"=w410:picture)
                  n80 = Select(t=w414, s=w413, f=w408) -> (s? t:f=w412:string)
                  n81 = Select(t=w411, s=w413, f=w410) -> (s? t:f=w409:picture)
                }
                frame "Running" {
                  w418 = "Running...!"  # Message
                  n82 = Unbundle By Name(w417) -> ("FlageData.BlueFlag"=w416:picture)
                }
                frame "FinishRunning" {
                  w421 = "Finish Line"  # Message
                  n83 = Unbundle By Name(w420) -> ("FlageData.CheckFlag"=w419:picture)
                }
                frame "DNF" {
                  w424 = "DNF"  # Message
                  n84 = Unbundle By Name(w423) -> ("FlageData.RedFlag"=w422:picture)
                }
              }
              n85 = case shown="\"Running\"" w365 {
                tunnel: [w387 w392 w396 w401 w404] -> w364
                tunnel: w363 -> [w386 w395 w398 w400 w403]
                tunnel: [w385 w389 w397 w399 w402] -> w362
                frame "Initial", Default {
                  w387 = "Initialize"  # Message
                  n86 = Unbundle By Name(w386) -> ("FlageData.RedFlag"=w385:picture)
                }
                frame "Ready" {
                  w388 = "Green Flag"  # Message
                  w394 = "Red Flag"  # Message
                  n87 = Unbundle By Name(w395) -> ("SignGreenFlag"=w393:bool, "FlageData.GreenFlag"=w391:picture, "FlageData.RedFlag"=w390:picture)
                  n88 = Select(t=w394, s=w393, f=w388) -> (s? t:f=w392:string)
                  n89 = Select(t=w391, s=w393, f=w390) -> (s? t:f=w389:picture)
                }
                frame "Running" {
                  w396 = "Running...!"  # Message
                  n90 = Unbundle By Name(w398) -> ("FlageData.BlueFlag"=w397:picture)
                }
                frame "FinishRunning" {
                  w401 = "Finish Line"  # Message
                  n91 = Unbundle By Name(w400) -> ("FlageData.CheckFlag"=w399:picture)
                }
                frame "DNF" {
                  w404 = "DNF"  # Message
                  n92 = Unbundle By Name(w403) -> ("FlageData.RedFlag"=w402:picture)
                }
              }
              n93 = call "IntegerTimeToLabTime.vi"("inputTime(msec)"=w378) -> ("outputTime(mm-ss-sss)"=w377:string)  [unwired: 10 in]
              n94 = call "IntegerTimeToLabTime.vi"("inputTime(msec)"=w380) -> ("outputTime(mm-ss-sss)"=w379:string)  [unwired: 10 in]
              n95 = Or Array Elements(Boolean array=w369) -> (logical OR=w370:bool)
              n96 = Or Array Elements(Boolean array=w367) -> (logical OR=w366:bool)
              n97 = And(x=w370, y=w366) -> (x .and. y?=w375:bool)
              n98 = Select(t=w381, s=w375, f=w376) -> (s? t:f=w382:T12)
              n99 = in-place-cluster #7("LapTime-A(ms)"=w378, "CurrentRecordIndicator.CurrentTime-A"=w377, "LapTime-B(ms)"=w380, "CurrentRecordIndicator.CurrentTime-B"=w379, "StateValue"=w382, "CurrentRecordIndicator.CurrentMessage-A"=w374, "CurrentRecordIndicator.Flag-A"=w373, "CurrentRecordIndicator.CurrentMessage-B"=w364, "CurrentRecordIndicator.Flag-B"=w362) -> (w349:T13)
            }
            n100 = call-poly <vilib>:"DAQmx Read.vi"("task/channels in"=w316, "error in"=w315) -> ("data"=w312:dbl[], "error out"=w308:errorcluster)  [unwired: 11 in, 1 out]
            n101 = Index Array(array=w312, index #1=w311) -> (element #1=w310:dbl, element #2=w309:dbl)  [unwired: 1 in]
            n102 = Unbundle By Name(w323) -> ("FlageData"=w322:T11, "SignRedFlag"=w314:bool, "SignGreenFlag"=w313:bool)
            n103 = call "DetectEdge(Analog).vi"("EdgeType"=w335, "Level(Voltage)"=w337, "Voltage"=w310) -> ("DetectedEdge"=w336:bool)  [unwired: 8 in]
            n104 = call "DetectEdge(Analog).vi"("EdgeType"=w334, "Level(Voltage)"=w338, "Voltage"=w309) -> ("DetectedEdge"=w330:bool)  [unwired: 8 in]
            n105 = in-place {
              in-place-border: w336 -> [w360]
              in-place-border: w323 -> [w361]
              n106 = in-place-cluster #8(w348) -> ()  [unwired: 4 out]
              n107 = Unbundle By Name(w361) -> ("SignGreenFlag"=w357:bool, "DNFEntry-A"=w359:bool, "RetryEntry-A"=w358:bool)
              n108 = in-place-cluster #8("PassLineEntry-A"=w360, "StartEntry-A"=w357, "DNFEntry-A"=w359, "RetryEntry-A"=w358) -> (w347:T9)
            }
            n109 = in-place {
              in-place-border: w330 -> [w355]
              in-place-border: w323 -> [w356]
              n110 = in-place-cluster #9(w331) -> ()  [unwired: 4 out]
              n111 = Unbundle By Name(w356) -> ("SignGreenFlag"=w352:bool, "DNFEntry-B"=w354:bool, "RetryEntry-B"=w353:bool)
              n112 = in-place-cluster #9("PassLineEntry-B"=w355, "StartEntry-B"=w352, "DNFEntry-B"=w354, "RetryEntry-B"=w353) -> (w329:T7)
            }
            n113 = Build Array(w314, w313, w314, w313) -> (w324:bool[])
            n114 = call "GymkhanaFlagSign.vi"("GreenFlagSignal"=w313, "RedFlagSignal"=w314, "inputFlageData"=w322) -> ("outputFlageData"=w321:T11)  [unwired: 8 in]
            n115 = Unbundle By Name(w321) -> ("RedFlag"=w319:picture, "GreenFlag"=w318:picture)
            n116 = call-poly <vilib>:"DAQmx Write.vi"("task/channels in"=w327, "data"=w324, "error in"=w326) -> ("error out"=w325:errorcluster)  [unwired: 10 in, 2 out]
            n117 = Bundle By Name(cluster=w320, "Red"=w319, "Green"=w318) -> (→"GymkhanaFlag":T1)
            n118 = Enqueue Element(queue=w351, element=w347, error in (no error)=w346) -> (error out=w344:errorcluster)  [unwired: 1 in, 2 out]
            n119 = Enqueue Element(queue=w350, element=w329, error in (no error)=w345) -> (error out=w343:errorcluster)  [unwired: 1 in, 2 out]
            n120 = Merge Errors "Merge Errors"(w332, w333, w328, w308, w325, w344, w343) -> (w342:errorcluster)
          }
          frame "RecordLog" {
            w426 = bool[] [FALSE, FALSE, FALSE, FALSE]  # data
            w431 = T1 {"Red"=bytes[0], "Blank"=bytes[0], "Green"=bytes[0]}  # GymkhanaFlag
            w441 = 3  # IndexColumn
            w440 = 0  # Index
            w452 = dbl[] [0.0, 0.0]  # data
            w463 = "LoggingData"  # SubFolderName
            w425 = FALSE
            w476 = TRUE  # append to file? (F)
            # "Logged File Format\nCurrentEntry <tab> CurrentUniversity <tab> CurrentTime(Display) <tab> 1LapTime(Absolute)"
            n121 = Unbundle By Name(w442) -> ("CurrentRecordIndicator.CurrentEntry-A"=w455:string, "CurrentRecordIndicator.CurrentUniversity-A"=w475:string, "CurrentRecordIndicator.CurrentTime-A"=w474:string, "CurrentRecordIndicator.CurrentEntry-B"=w454:string, "CurrentRecordIndicator.CurrentUniversity-B"=w468:string, "CurrentRecordIndicator.CurrentTime-B"=w467:string, "LapTime-A(ms)"=w460:i64, "LapTime-B(ms)"=w458:i64)
            n122 = call-poly <vilib>:"DAQmx Write.vi"("task/channels in"=w450, "data"=w452, "error in"=w451) -> ("task out"=w449:refnum<k21>, "error out"=w448:errorcluster)  [unwired: 10 in, 1 out]
            n123 = call-poly <vilib>:"DAQmx Write.vi"("task/channels in"=w430, "data"=w426, "error in"=w429) -> ("task out"=w428:refnum<k21>, "error out"=w427:errorcluster)  [unwired: 10 in, 1 out]
            n124 = call <vilib>:"DAQmx Stop Task.vi"("task/channels in"=w449, "error in"=w448) -> ("error out"=w447:errorcluster)  [unwired: 12 in, 1 out]
            n125 = call <vilib>:"DAQmx Stop Task.vi"("task/channels in"=w446, "error in"=w445) -> ("error out"=w444:errorcluster)  [unwired: 12 in, 1 out]
            n126 = call <vilib>:"DAQmx Stop Task.vi"("task/channels in"=w428, "error in"=w427) -> ("error out"=w432:errorcluster)  [unwired: 12 in, 1 out]
            n127 = Number To Decimal String(number=w460) -> (decimal integer string=w459:string)  [unwired: 1 in]
            n128 = Number To Decimal String(number=w458) -> (decimal integer string=w457:string)  [unwired: 1 in]
            n129 = Concatenate Strings "Concatenate Strings"(w455, w454) -> (w453:string)
            n130 = Current VI's Path() -> (path=w462:path)
            n131 = Build Array(w454, w468, w467, w457) -> (w469:string[])
            n132 = Build Array(w455, w475, w474, w459) -> (w471:string[])
            n133 = call "ScreenShotFrontPannel.vi"("SubFolderName"=w463, "FileName"=w453, "vi path"=w462) -> ("error out"=w461:errorcluster)  [unwired: 8 in]
            n134 = Build Array "Build Array"(w471, w469) -> (w470:string[][])
            n135 = for {
              tunnel: w476 -> [w486]
              tunnel: w472 -> [w483]
              shift-right: [w485] -> w438
              shift-left: w473 -> [w484]
              tunnel: w470 -> [w482] mode=indexing
              tunnel: [w481] -> w439
              n136 = call-poly <vilib>:"Write Delimited Spreadsheet.vi"("file path (dialog if empty)"=w483, "1D data"=w482, "append to file? (new file:F)"=w486, "error in (no error)"=w484) -> ("new file path (Not A Path if cancelled)"=w481:path, "error out"=w485:errorcluster)  [unwired: 10 in]
            }
            n137 = call "ReadBestRecord.vi"("IndexColumn"=w441, "ErrorInput"=w438, "FilepathInput"=w439) -> ("ErrorOutput"=w437:errorcluster, "Data"=w436:string[])  [unwired: 6 in, 1 out]
            n138 = Index Array "Index Array"(array=w436, index #1=w440) -> (element #1=w435:string, element #2=w434:string, element #3=w433:string)  [unwired: 2 in]
            n139 = local write "GreenFlag"(w425) -> ()
            n140 = local write "RedFlag"(w425) -> ()
            n141 = local write "GymkhanaFlag"(w431) -> ()
            n142 = in-place {
              in-place-border: w435 -> [w480]
              in-place-border: w434 -> [w479]
              in-place-border: w433 -> [w478]
              w477 = GymkhanaMainLoopState."WaittingforNext"  # GymkhanaMainLoopState
              n143 = in-place-cluster #10(w442) -> ()  [unwired: 4 out]
              n144 = in-place-cluster #10("StateValue"=w477, "BestRecordIndicator.BestEntry"=w480, "BestRecordIndicator.BestUniv"=w479, "BestRecordIndicator.BestTime"=w478) -> (w443:T13)
            }
            n145 = Merge Errors "Merge Errors"(w456, w437, w461, w447, w444, w432, w466, w465) -> (w464:errorcluster)
          }
          frame "WaittingforNext" {
            w497 = GymkhanaSubLoopState."Ready"  # GymkhanaSubLooptate
            n146 = Unbundle By Name(w498) -> ("GymkhanaSubLooptate"=w491:T2)
            n147 = Unbundle By Name(w499) -> ("GymkhanaSubloopState"=w492:T2)
            n148 = in-place {
              in-place-border: w500 -> [w517]
              n149 = in-place-cluster #11(w505) -> ()  [unwired: 1 out]
              n150 = Unbundle By Name(w517) -> ("NextEntry"=w516:bool)
              n151 = in-place-cluster #11("NextEntry-A"=w516) -> (w503:T9)
            }
            n152 = in-place {
              in-place-border: w500 -> [w515]
              n153 = in-place-cluster #12(w504) -> ()  [unwired: 1 out]
              n154 = Unbundle By Name(w515) -> ("NextEntry"=w514:bool)
              n155 = in-place-cluster #12("NextEntry-B"=w514) -> (w502:T7)
            }
            n156 = Build Array(w492, w491) -> (w490:T2[])
            n157 = Equal?(x=w497, y=w490) -> (x = y?=w489:bool[])
            n158 = And Array Elements(Boolean array=w489) -> (logical AND=w496:bool)
            n159 = Enqueue Element(queue=w513, element=w503, error in (no error)=w512) -> (error out=w509:errorcluster)  [unwired: 1 in, 2 out]
            n160 = Enqueue Element(queue=w511, element=w502, error in (no error)=w510) -> (error out=w508:errorcluster)  [unwired: 1 in, 2 out]
            n161 = in-place {
              in-place-border: w496 -> [w521]
              w518 = GymkhanaMainLoopState."Initial"  # t
              n162 = in-place-cluster #13(w500) -> ("StateValue"=w520:T12)
              n163 = Select(t=w518, s=w521, f=w520) -> (s? t:f=w519:T12)
              n164 = in-place-cluster #13("StateValue"=w519) -> (w506:T13)
            }
            n165 = Merge Errors "Merge Errors"(w493, w488, w495, w494, w487, w509, w508) -> (w507:errorcluster)
          }
          frame "ProgramStop" {
            w541 = dbl[] [0.0, 0.0]  # data
            n166 = call <vilib>:"DAQmx Stop Task.vi"("task/channels in"=w534, "error in"=w535) -> ("task out"=w539:refnum<k21>, "error out"=w538:errorcluster)  [unwired: 12 in]
            n167 = call <vilib>:"DAQmx Stop Task.vi"("task/channels in"=w524, "error in"=w523) -> ("task out"=w525:refnum<k21>, "error out"=w526:errorcluster)  [unwired: 12 in]
            n168 = Release Queue(queue=w551, error in (no error)=w550) -> (error out=w533:errorcluster)  [unwired: 1 in, 2 out]
            n169 = Release Queue(queue=w549, error in (no error)=w548) -> (error out=w532:errorcluster)  [unwired: 1 in, 2 out]
            n170 = in-place {
              in-place-border: w545 -> [w553]
              w554 = "Halted Program"  # CurrentRecordIndicator.CurrentMessage-A
              n171 = in-place-cluster #14(w545) -> ()  [unwired: 4 out]
              n172 = Unbundle By Name(w553) -> ("FlageData.RedFlag"=w552:picture)
              n173 = in-place-cluster #14("CurrentRecordIndicator.Flag-A"=w552, "CurrentRecordIndicator.Flag-B"=w552, "CurrentRecordIndicator.CurrentMessage-A"=w554, "CurrentRecordIndicator.CurrentMessage-B"=w554) -> (w546:T13)
            }
            n174 = call <vilib>:"DAQmx Clear Task.vi"("task in"=w539, "error in"=w538) -> ("error out"=w537:errorcluster)  [unwired: 13 in]
            n175 = call <vilib>:"DAQmx Clear Task.vi"("task in"=w525, "error in"=w526) -> ("error out"=w522:errorcluster)  [unwired: 13 in]
            n176 = call-poly <vilib>:"DAQmx Write.vi"("task/channels in"=w530, "data"=w541, "error in"=w529) -> ("task out"=w543:refnum<k21>, "error out"=w542:errorcluster)  [unwired: 10 in, 1 out]
            n177 = call <vilib>:"DAQmx Stop Task.vi"("task/channels in"=w543, "error in"=w542) -> ("task out"=w544:refnum<k21>, "error out"=w540:errorcluster)  [unwired: 12 in]
            n178 = call <vilib>:"DAQmx Clear Task.vi"("task in"=w544, "error in"=w540) -> ("error out"=w536:errorcluster)  [unwired: 13 in]
            n179 = Merge Errors "Merge Errors"(w527, w528, w536, w537, w522, w533, w532) -> (w531:errorcluster)
          }
        }
        n180 = in-place {
          in-place-border: w199 -> [w560]
          in-place-border: w196 -> [w557]
          w559 = GymkhanaMainLoopState."ProgramStop"  # t
          n181 = in-place-cluster #15(w196) -> ("StateValue"=w555:T12)
          n182 = Unbundle By Name(w557) -> ("Stop"=w556:bool)
          n183 = Or(x=w556, y=w560) -> (x .or. y?=w561:bool)
          n184 = Select(t=w559, s=w561, f=w555) -> (s? t:f=w558:T12)
          n185 = in-place-cluster #15("StateValue"=w558) -> (w202:T13)
        }
        n186 = Unbundle By Name(w202) -> ("CurrentRecordIndicator"=→"CurrentRecordIndicator":T5, "BestRecordIndicator"=→"BestRecordIndicator":T6)
        n187 = Wait Until Next ms Multiple(millisecond multiple=w220) -> ()  [unwired: 1 out]
      }
      n188 = while {
        tunnel: w115 -> [w577]
        tunnel: w112 -> [w576]
        shift-right: [w569] -> _
        shift-left: w106 -> [w570]
        stop <- w575 stop-if-true
        # "Entry A LabTime"
        n189 = Dequeue Element(queue=w577, error in (no error)=w576) -> (element=w571:T9, error out=w575:errorcluster)  [unwired: 1 in, 2 out]
        n190 = Unbundle By Name(w571) -> ("DNFEntry-A"=w568:bool, "RetryEntry-A"=w565:bool, "StartEntry-A"=w564:bool, "PassLineEntry-A"=w563:bool, "NextEntry-A"=w562:bool)
        n191 = in-place {
          in-place-border: w568 -> [w583]
          n192 = in-place-cluster #16(w570) -> ("GymkhanaSubloopState"=w587:T2, "Entry-A-LabTime(ms)"=w585:i64)
          n193 = call "GymkhanaDNFRoll.vi"("inputDNF"=w583, "inputLabTIme(ms)"=w585, "inputGymkhanaSubLooptate"=w587) -> ("outputLabTime(ms)"=w584:i64, "outputGymkhanaSubLooptate"=w586:T2)  [unwired: 7 in]
          n194 = in-place-cluster #16("GymkhanaSubloopState"=w586, "Entry-A-LabTime(ms)"=w584) -> (w567:T8)
        }
        n195 = in-place {
          in-place-border: w565 -> [w578]
          n196 = in-place-cluster #17(w567) -> ("GymkhanaSubloopState"=w582:T2, "Entry-A-LabTime(ms)"=w580:i64)
          n197 = call "GymkhanaRetryRoll.vi"("inputRetry"=w578, "inputLabTIme(ms)"=w580, "inputGymkhanaSubLooptate"=w582) -> ("outputLabTime(ms)"=w579:i64, "outputGymkhanaSubLooptate"=w581:T2)  [unwired: 7 in]
          n198 = in-place-cluster #17("GymkhanaSubloopState"=w581, "Entry-A-LabTime(ms)"=w579) -> (w566:T8)
        }
        n199 = Unbundle By Name(w566) -> ("GymkhanaSubloopState"=w572:T2)
        n200 = Tick Count (ms)() -> (millisecond timer value=w574:u32)
        n201 = To Quad Integer(1:w574) -> (0:w573:i64)
        n202 = case shown="\"Running\"" w572 {
          tunnel: w573 -> [_ w595 w604 _ _]
          tunnel: w566 -> [w589 w596 w605 w618 w625]
          tunnel: [w588 w594 w603 w617 w624] -> w569
          tunnel: w564 -> [_ w593 _ _ _]
          tunnel: w563 -> [_ w592 w602 _ _]
          tunnel: w562 -> [_ _ _ w616 w623]
          frame "Initial", Default {
            n203 = in-place {
              w590 = GymkhanaSubLoopState."Ready"  # GymkhanaSubloopState
              w591 = i64 0  # Entry-ARefTime(ms)
              n204 = in-place-cluster #18(w589) -> ()  [unwired: 3 out]
              n205 = in-place-cluster #18("Entry-A-RefTime(ms)"=w591, "Entry-A-LabTime(ms)"=w591, "GymkhanaSubloopState"=w590) -> (w588:T8)
            }
          }
          frame "Ready" {
            n206 = in-place {
              in-place-border: w595 -> [w601]
              in-place-border: w593 -> [w597]
              in-place-border: w592 -> [_]
              w599 = GymkhanaSubLoopState."Running"  # t
              n207 = in-place-cluster #19(w596) -> ("GymkhanaSubloopState"=w598:T2)  [unwired: 1 out]
              n208 = Select(t=w599, s=w597, f=w598) -> (s? t:f=w600:T2)
              n209 = in-place-cluster #19("Entry-A-RefTime(ms)"=w601, "GymkhanaSubloopState"=w600) -> (w594:T8)
            }
          }
          frame "Running" {
            n210 = in-place {
              in-place-border: w604 -> [w613]
              in-place-border: w602 -> [w606]
              w612 = i64 3000  # y
              w615 = GymkhanaSubLoopState."FinishRunning"  # t
              n211 = in-place-cluster #20(w605) -> ("Entry-A-RefTime(ms)"=w614:i64, "GymkhanaSubloopState"=w610:T2)  [unwired: 1 out]
              n212 = Subtract(x=w613, y=w614) -> (x-y=w607:i64)
              n213 = Greater Or Equal?(x=w607, y=w612) -> (x >= y?=w611:bool)
              n214 = And(x=w611, y=w606) -> (x .and. y?=w608:bool)
              n215 = Select(t=w615, s=w608, f=w610) -> (s? t:f=w609:T2)
              n216 = in-place-cluster #20("Entry-A-RefTime(ms)"=w614, "Entry-A-LabTime(ms)"=w607, "GymkhanaSubloopState"=w609) -> (w603:T8)
            }
          }
          frame "DNF" {
            n217 = in-place {
              in-place-border: w616 -> [w622]
              w619 = GymkhanaSubLoopState."Initial"  # t
              n218 = in-place-cluster #21(w618) -> ("GymkhanaSubloopState"=w620:T2)
              n219 = Select(t=w619, s=w622, f=w620) -> (s? t:f=w621:T2)
              n220 = in-place-cluster #21("GymkhanaSubloopState"=w621) -> (w617:T8)
            }
          }
          frame "FinishRunning" {
            n221 = in-place {
              in-place-border: w623 -> [w626]
              w627 = GymkhanaSubLoopState."Initial"  # t
              n222 = in-place-cluster #22(w625) -> ("GymkhanaSubloopState"=w629:T2)
              n223 = Select(t=w627, s=w626, f=w629) -> (s? t:f=w628:T2)
              n224 = in-place-cluster #22("GymkhanaSubloopState"=w628) -> (w624:T8)
            }
          }
        }
        "Entry-A-InternalData" <- w569
      }
      n225 = while {
        tunnel: w103 -> [w140]
        tunnel: w104 -> [w139]
        shift-right: [w132] -> _
        shift-left: w105 -> [w133]
        stop <- w138 stop-if-true
        # "Entry A LabTime"
        n226 = Dequeue Element(queue=w140, error in (no error)=w139) -> (element=w134:T7, error out=w138:errorcluster)  [unwired: 1 in, 2 out]
        n227 = Unbundle By Name(w134) -> ("DNFEntry-B"=w131:bool, "RetryEntry-B"=w128:bool, "StartEntry-B"=w127:bool, "PassLineEntry-B"=w126:bool, "NextEntry-B"=w125:bool)
        n228 = in-place {
          in-place-border: w131 -> [w146]
          n229 = in-place-cluster #23(w133) -> ("GymkhanaSubLooptate"=w150:T2, "Entry-B-LabTime(ms)"=w148:i64)
          n230 = call "GymkhanaDNFRoll.vi"("inputDNF"=w146, "inputLabTIme(ms)"=w148, "inputGymkhanaSubLooptate"=w150) -> ("outputLabTime(ms)"=w147:i64, "outputGymkhanaSubLooptate"=w149:T2)  [unwired: 7 in]
          n231 = in-place-cluster #23("GymkhanaSubLooptate"=w149, "Entry-B-LabTime(ms)"=w147) -> (w130:T3)
        }
        n232 = in-place {
          in-place-border: w128 -> [w141]
          n233 = in-place-cluster #24(w130) -> ("GymkhanaSubLooptate"=w145:T2, "Entry-B-LabTime(ms)"=w143:i64)
          n234 = call "GymkhanaRetryRoll.vi"("inputRetry"=w141, "inputLabTIme(ms)"=w143, "inputGymkhanaSubLooptate"=w145) -> ("outputLabTime(ms)"=w142:i64, "outputGymkhanaSubLooptate"=w144:T2)  [unwired: 7 in]
          n235 = in-place-cluster #24("GymkhanaSubLooptate"=w144, "Entry-B-LabTime(ms)"=w142) -> (w129:T3)
        }
        n236 = Unbundle By Name(w129) -> ("GymkhanaSubLooptate"=w135:T2)
        n237 = Tick Count (ms)() -> (millisecond timer value=w137:u32)
        n238 = To Quad Integer(1:w137) -> (0:w136:i64)
        n239 = case shown="\"Running\"" w135 {
          tunnel: w136 -> [_ w158 w167 _ _]
          tunnel: w129 -> [w152 w159 w168 w181 w188]
          tunnel: [w151 w157 w166 w180 w186] -> w132
          tunnel: w127 -> [_ w156 _ _ _]
          tunnel: w126 -> [_ w155 w165 _ _]
          tunnel: w125 -> [_ _ _ w179 w187]
          frame "Initial", Default {
            n240 = in-place {
              w153 = GymkhanaSubLoopState."Ready"  # GymkhanaSubloopState
              w154 = i64 0  # Entry-ARefTime(ms)
              n241 = in-place-cluster #25(w152) -> ()  [unwired: 3 out]
              n242 = in-place-cluster #25("Entry-B-RefTime(ms)"=w154, "Entry-B-LabTime(ms)"=w154, "GymkhanaSubLooptate"=w153) -> (w151:T3)
            }
          }
          frame "Ready" {
            n243 = in-place {
              in-place-border: w158 -> [w164]
              in-place-border: w156 -> [w160]
              in-place-border: w155 -> [_]
              w162 = GymkhanaSubLoopState."Running"  # t
              n244 = in-place-cluster #26(w159) -> ("GymkhanaSubLooptate"=w161:T2)  [unwired: 1 out]
              n245 = Select(t=w162, s=w160, f=w161) -> (s? t:f=w163:T2)
              n246 = in-place-cluster #26("Entry-B-RefTime(ms)"=w164, "GymkhanaSubLooptate"=w163) -> (w157:T3)
            }
          }
          frame "Running" {
            n247 = in-place {
              in-place-border: w167 -> [w176]
              in-place-border: w165 -> [w169]
              w175 = i64 3000  # y
              w178 = GymkhanaSubLoopState."FinishRunning"  # t
              n248 = in-place-cluster #27(w168) -> ("Entry-B-RefTime(ms)"=w177:i64, "GymkhanaSubLooptate"=w173:T2)  [unwired: 1 out]
              n249 = Subtract(x=w176, y=w177) -> (x-y=w170:i64)
              n250 = Greater Or Equal?(x=w170, y=w175) -> (x >= y?=w174:bool)
              n251 = And(x=w174, y=w169) -> (x .and. y?=w171:bool)
              n252 = Select(t=w178, s=w171, f=w173) -> (s? t:f=w172:T2)
              n253 = in-place-cluster #27("Entry-B-RefTime(ms)"=w177, "Entry-B-LabTime(ms)"=w170, "GymkhanaSubLooptate"=w172) -> (w166:T3)
            }
          }
          frame "FinishRunning" {
            n254 = in-place {
              in-place-border: w179 -> [w182]
              w183 = GymkhanaSubLoopState."Initial"  # t
              n255 = in-place-cluster #28(w181) -> ("GymkhanaSubLooptate"=w185:T2)
              n256 = Select(t=w183, s=w182, f=w185) -> (s? t:f=w184:T2)
              n257 = in-place-cluster #28("GymkhanaSubLooptate"=w184) -> (w180:T3)
            }
          }
          frame "DNF" {
            n258 = in-place {
              in-place-border: w187 -> [w192]
              w189 = GymkhanaSubLoopState."Initial"  # t
              n259 = in-place-cluster #29(w188) -> ("GymkhanaSubLooptate"=w190:T2)
              n260 = Select(t=w189, s=w192, f=w190) -> (s? t:f=w191:T2)
              n261 = in-place-cluster #29("GymkhanaSubLooptate"=w191) -> (w186:T3)
            }
          }
        }
        "Entry-B-InternalData" <- w132
      }
    }
    frame #2 {
      n262 = call <vilib>:"Simple Error Handler.vi"("error in (no error)"=w630) -> ()  [unwired: 4 in, 5 out]
    }
  }
  n263 = flat-sequence {
    frame #0 {
      # "Finalized"
      n264 = call <vilib>:"Simple Error Handler.vi"() -> ()  [unwired: 5 in, 5 out]
    }
  }
